vi "Main.vi"() -> ()   [LabVIEW 2019]
doc: "This Continuous Measurement sample project is based on the Queued Message Handler template.\n\nThe Event Handling Loop generates messages based on user interface actions.\n\nThe Message Handling Loop processes messages generated by the Event Handling Loop, or by other messages. There are also Acquisition and Logging message handling loop subVIs, and a chart updating loop."
uses:
  Settings/Settings.ctl
  HardwareAdapter/Support/Hardware Configuration.ctl
  HardwareAdapter/Support/Camera Configuration.ctl
  D:/SDK/PMQI-LabViewSamples/Examples/Dependencies/PVCamNET.dll
  <vilib>/userdefined/High Color/IMAQdx.ctl
  E:/DevHardSoftware/MMicroscopy/HardwareAdapter/Lasers/Dependencies/Oxxius_Boxx.dll
  HardwareAdapter/Lasers/Dependencies/Oxxius_Boxx.dll
  Logging/Logging Configuration.ctl
  controls/UI Configuration.ctl
  controls/CallBack Refs.ctl
  controls/UI Data.ctl
  controls/UI State.ctl
  controls/ImageInfo.ctl
  <vilib>/vision/Image Controls.llb/IMAQ Image.ctl
  HardwareAdapter/Lasers/Laser Ctrl.ctl
  HardwareAdapter/Stages/Stage Ctrl.ctl
  Global.vi
  support/Message Queue/Enqueue Message (Single).vi
  <vilib>/Utility/error.llb/Error Cluster From Error Code.vi
  <vilib>/ErrorRing/Error Ring.xnode
  Acquisition/Acquisition.lvlib
  Logging/Logging.lvlib
  Settings/Settings.lvlib
  support/User Event - Stop/User Event - Stop.lvlib
  support/Message Queue/Message Queue.lvlib
  Settings/Settings Dialog.vi
panel:
  in  "DropFrame":dbl
  in  "FrameIndexSroll":i32(c297)
  in  "RealFPS":dbl
  in  "FrameRate":dbl
  in  "CaptureFrame":dbl
  in  "Exposure":dbl
  in  "CurrentFrame":dbl
  out "CapturingLED":bool caption="Capturing"
  in  "TableTap":T1(tab)
  out "8 Bit Histogram":u32[](graph)
  out "EPILimit":bool
  out "TIRFLimit":bool
  in  "MicroStage+":dbl
  in  "TIRF-":bool
  in  "TIRF--":bool
  in  "EPI++":bool
  in  "EPI+":bool
  out "TirfModuleScollBar":u8(slide) scale=0.0..100.0
  in  "Anti-Drifft XY":bool
  out "NanoStage X":dbl(graph)
  out "NanoStage  Y":dbl(graph)
  out "NanoStage Z":dbl(graph)
  out "TIRF-Lock":cluster{"X":dbl, "Y":dbl}[](graph)
  in  "TIRF-Lock Z":bool
  in  "StageX-":bool
  in  "StageX+":bool
  in  "StageY+":bool
  in  "StageY-":bool
  in  "StageZ++":bool
  in  "StageZ--":bool
  in  "StageY++":bool
  in  "StageZ+":bool
  in  "StageZ-":bool
  in  "StageX--":bool
  in  "StageX++":bool
  in  "StageY--":bool
  in  "XYIncreatement+":dbl
  in  "XYIncreatement++":dbl
  in  "ZIncreatement+":dbl
  in  "ZIncreatement++":dbl
  in  "TIRF-LockCalbrate":bool
  out "Min":u32
  out "Max":u32
  out "Mean":dbl
  in  "FileSaveButton":bool
  in  "NoteAutoSave":bool caption="AutoSave"
  in  "Note":string
  in  "FilePrefix":string
  in  "Config":T2 {"Hardware Configuration"."Lasers Configuration"."SettingValues"."785 Power" format="%.1f"; "Hardware Configuration"."Lasers Configuration"."SettingValues"."647 Power" format="%.1f"; "Hardware Configuration"."Lasers Configuration"."SettingValues"."561 Power" format="%.1f"; "Hardware Configuration"."Lasers Configuration"."SettingValues"."532 Power" format="%.1f"; "Hardware Configuration"."Lasers Configuration"."SettingValues"."488 Power" format="%.1f"; "Hardware Configuration"."Lasers Configuration"."SettingValues"."405 Power" format="%.1f"}
  in  "Save Settings":bool
  in  "AutoFocus":bool
  in  "AddROI":bool
  in  "Record":bool
  in  "Power785":dbl
  in  "785 nm":bool
  in  "Power647":sgl
  in  "647 nm":bool
  in  "Power561":dbl
  in  "561 nm":bool
  in  "Power532":sgl
  in  "532 nm":bool
  in  "Power488":dbl
  in  "488 nm":bool
  in  "Power405":dbl
  in  "405 nm":bool
  out "DeviceStatus":T9
  out "Status":string
  in  "Exit":bool
  in  "Settings":bool
  in  "Stop":bool
  in  "Album":bool
  out "RecordLED":bool caption="Rec"
  out "LiveLED":bool caption="Live"
  out "RawImage":T10(plugin-control)
  # "Power(%)"
  # "On"
  # "Off"
  # "Lasers"
  # "Y"
  # "μm"
  # "μm"
  # "μm"
  # "μm"
  # "X"
  # "TIRF"
  # "EPI"
  # "Z"
  # "μm"
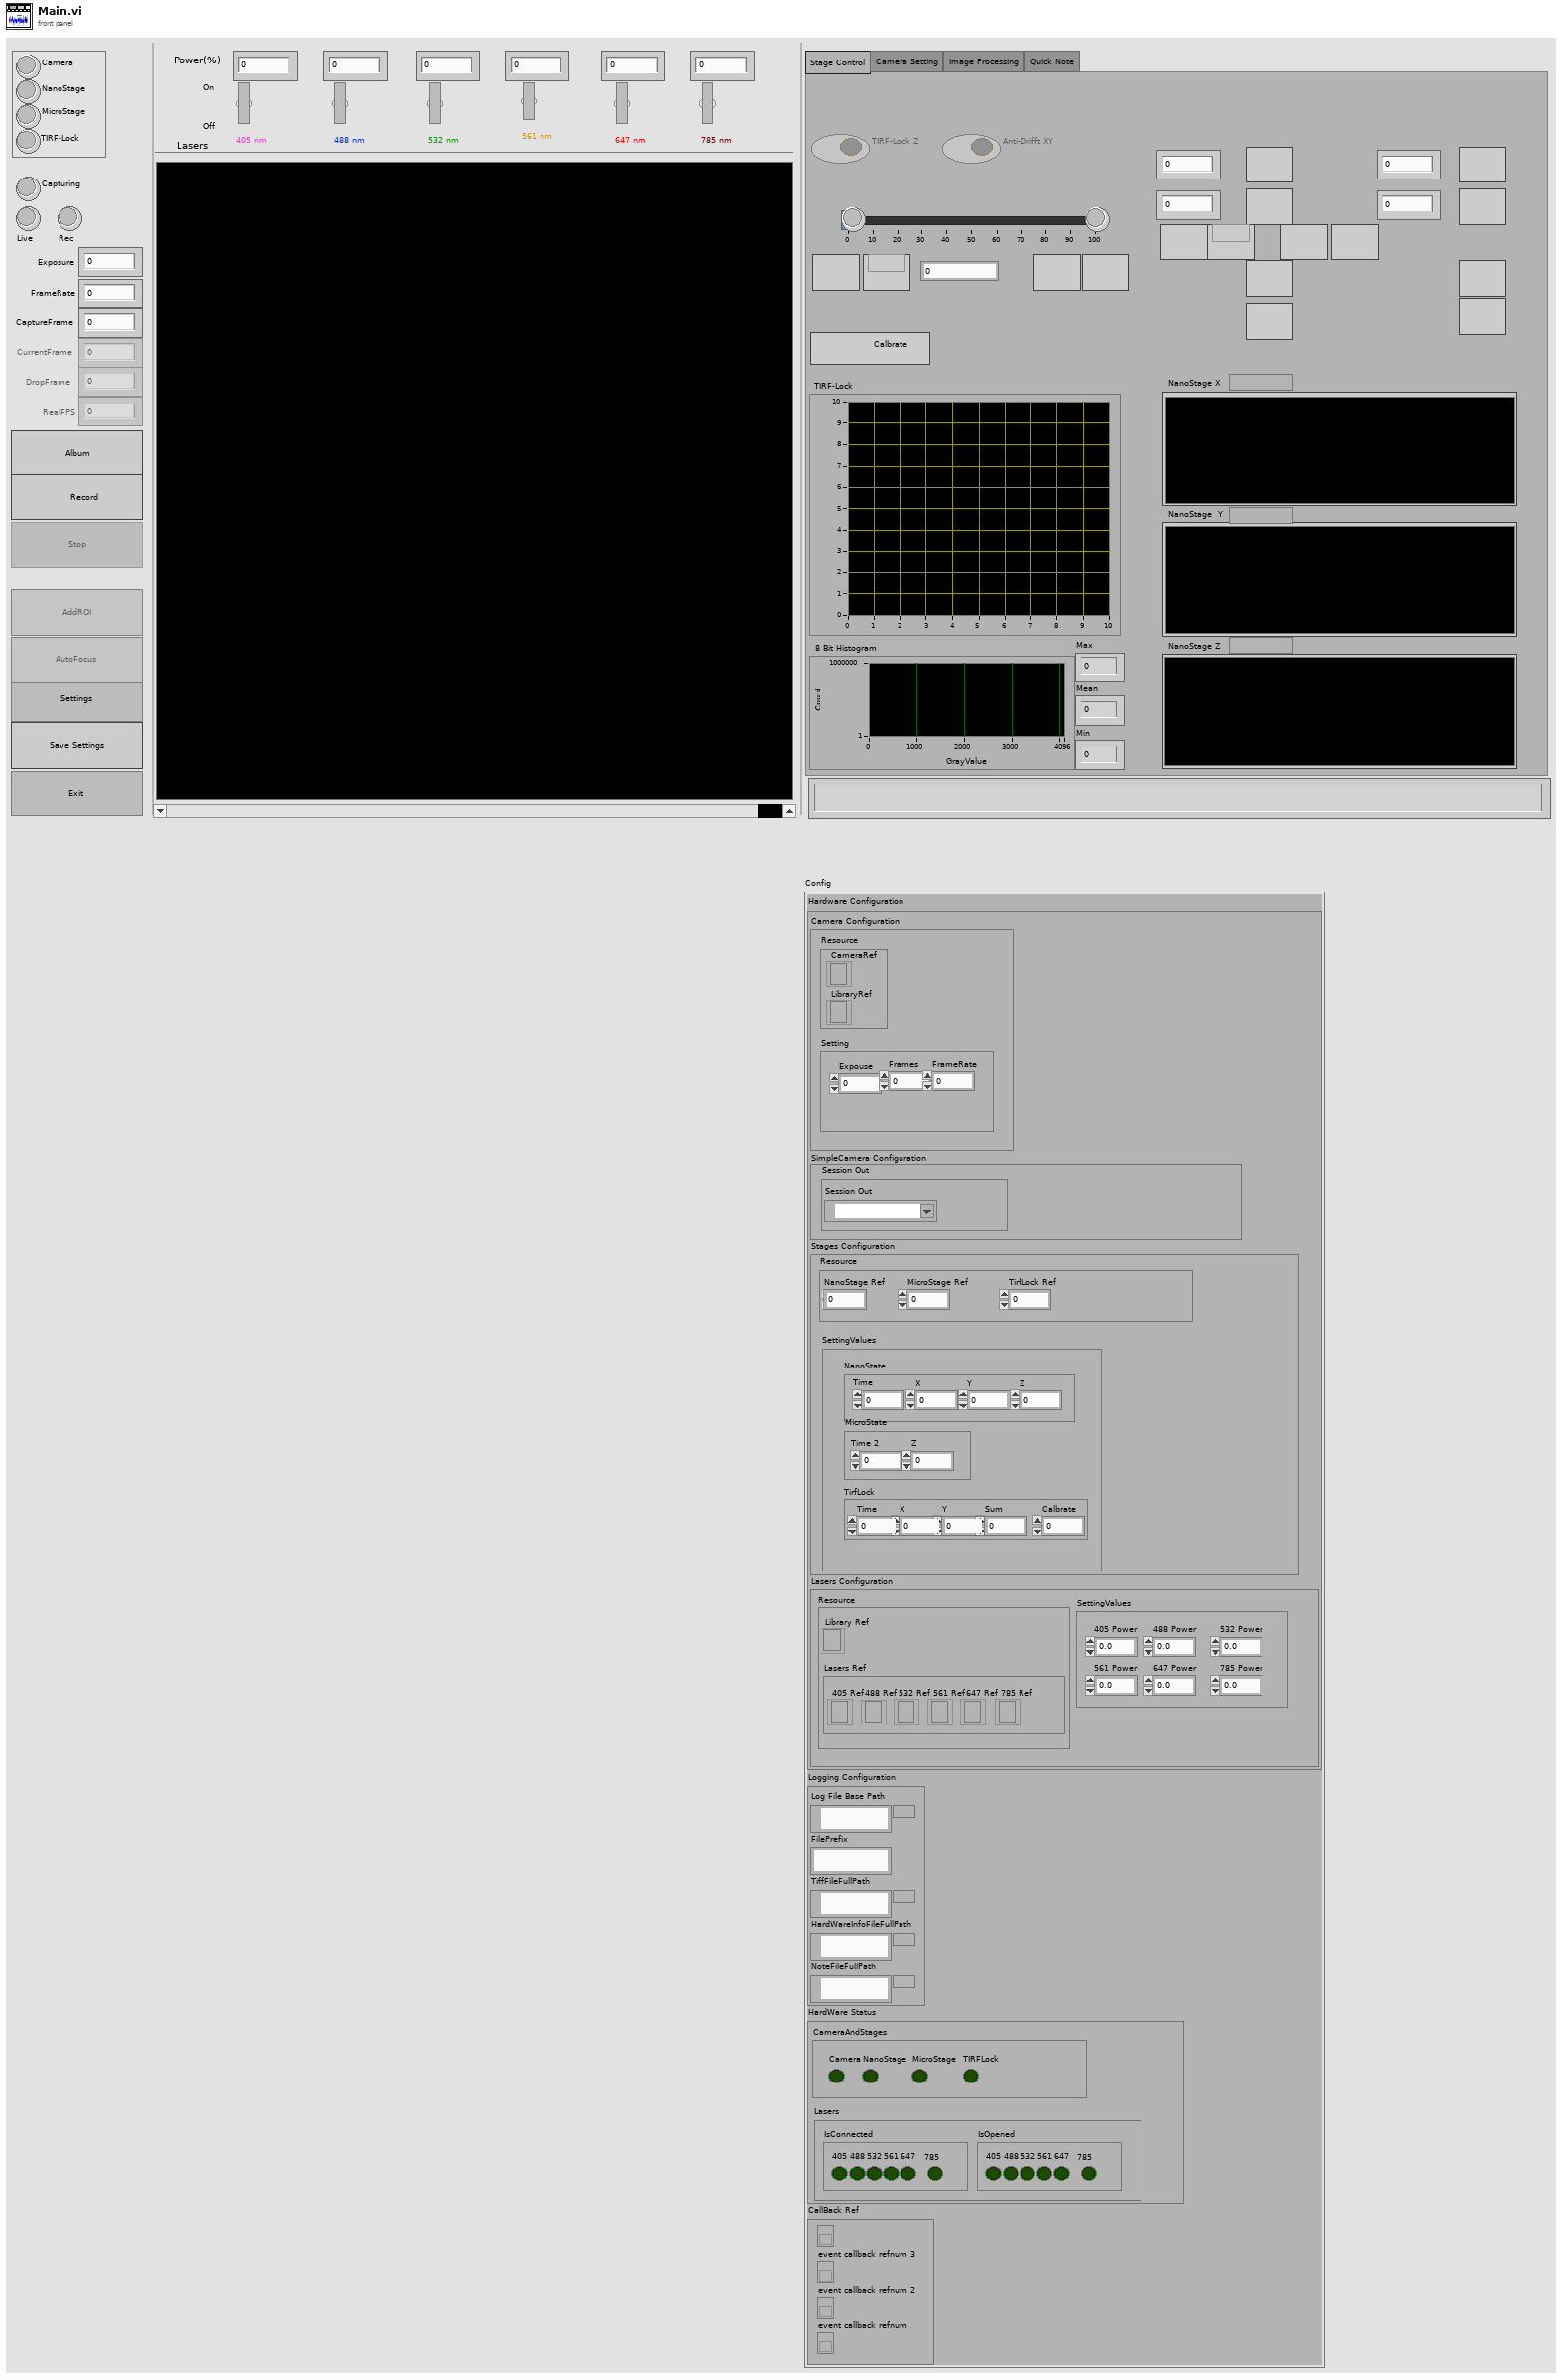
[diagram p1: front panel]
types:
  T1 = enum32{"Stage Control", "Camera Setting", "Image Processing", "Quick Note"}
  T2 = typedef "Settings.lvlib/Settings.ctl" = cluster{"Hardware Configuration":T3, "Logging Configuration":T6, "HardWare Status":cluster{"CameraAndStages":T7, "Lasers":cluster{"IsConnected":cluster{"405":bool, "488":bool, "532":bool, "561":bool, "647":bool, "785":bool}, "IsOpened":cluster{"405":bool, "488":bool, "532":bool, "561":bool, "647":bool, "785":bool}}}, "CallBack Ref":T8}
  T3 = typedef "Hardware Configuration.ctl" = cluster{"Camera Configuration":T4, "SimpleCamera Configuration":cluster{"Resource":cluster{"Session Out":T5}}, "Stages Configuration":cluster{"Resource":cluster{"NanoStage Ref":i32, "MicroStage Ref":i32, "TirfLock Ref":i32}, "SettingValues":cluster{"NanoState":cluster{"Time":dbl, "X":dbl, "Y":dbl, "Z":dbl}, "MicroState":cluster{"Time 2":dbl, "Z":dbl}, "TirfLock":cluster{"Time":dbl, "X":dbl, "Y":dbl, "Sum":dbl, "Calbrate":dbl}}}, "Lasers Configuration":cluster{"SettingValues":cluster{"405 Power":sgl, "488 Power":sgl, "532 Power":sgl, "561 Power":sgl, "647 Power":sgl, "785 Power":sgl}, "Resource":cluster{"Library Ref":refnum<k24>, "Lasers Ref":cluster{"405 Ref":refnum<k24>, "488 Ref":refnum<k24>, "532 Ref":refnum<k24>, "561 Ref":refnum<k24>, "647 Ref":refnum<k24>, "785 Ref":refnum<k24>}}}}
  T4 = typedef "Camera Configuration.ctl" = cluster{"Resource":cluster{"CameraRef":refnum<k24>, "LibraryRef":refnum<k24>}, "Setting":cluster{"Expouse":dbl, "Frames":dbl, "FrameRate":dbl}}
  T5 = typedef "IMAQdx.ctl" = refnum<k21>
  T6 = typedef "Logging.lvlib/Logging Configuration.ctl" = cluster{"Log File Base Path":path, "FilePrefix":string, "TiffFileFullPath":path, "HardWareInfoFileFullPath":path, "NoteFileFullPath":path}
  T7 = typedef "UI Configuration.ctl" = cluster{"Camera":bool, "NanoStage":bool, "MicroStage":bool, "TIRFLock":bool}
  T8 = typedef "CallBack Refs.ctl" = cluster{"event callback refnum":refnum<k27>, "event callback refnum 2":refnum<k27>, "event callback refnum 3":refnum<k27>, "event callback refnum 4":refnum<k27>}
  T9 = cluster{"Camera":bool, "NanoStage":bool, "MicroStage":bool, "TIRF-Lock":bool}
  T10 = typedef "IMAQ Image.ctl" = refnum<image>
  T11 = typedef "UI State.ctl" = enum16{"Idle", "Acquiring and Logging", "Waiting for Exit", "Waiting for Exit (Acq Stopped)", "Waiting for Exit (Ctrl Stopped)", "Waiting for Exit (Log Stopped)", "Waiting for Stop", "Waiting for Stop (Acq Stopped)", "Waiting for Stop (Ctrl Stopped)", "Waiting for Stop (Log Stopped)"}
  T12 = typedef "UI Data.ctl" = cluster{"Album Ref":refnum<vi>, "Stop Ref":refnum<vi>, "Settings Ref":refnum<vi>, "Exit Ref":refnum<vi>, "Status Ref":refnum<vi>, "Record Ref":refnum<vi>, "785 Ref":refnum<vi>, "647 Ref":refnum<vi>, "532 Ref":refnum<vi>, "561 Ref":refnum<vi>, "488 Ref":refnum<vi>, "405 Ref":refnum<vi>, "Power561 Ref":refnum<vi>, "Power405 Ref":refnum<vi>, "Power488 Ref":refnum<vi>, "Power785 Ref":refnum<vi>, "Power532 Ref":refnum<vi>, "Power647 Ref":refnum<vi>, "TIRFLock Ref":refnum<vi>, "AntiDrifft Ref":refnum<vi>, "Histogram":refnum<vi>, "Capturing":refnum<vi>, "FrameIndex":refnum<vi>, "RealFPS":refnum<vi>, "FrameIndexSroll":refnum<vi>, "DropFrame":refnum<vi>}
  T13 = typedef "Message Queue.lvlib/All Message Queues.ctl" = cluster{"UI":refnum<queue>, "Acquisition":refnum<queue>, "Logging":refnum<queue>, "Control":refnum<queue>}
  T14 = typedef "DataQueuesAndNotifier.ctl" = cluster{"DataQueues":refnum<queue>[], "DataNotifier":refnum<notifier>[]}
  T15 = typedef "ImageInfo.ctl" = cluster{"Time":dbl, "Image":T10, "Histogram":u32[], "MeanValue":dbl, "Min":u32, "Max":u32}
  T16 = typedef "LVPoint32TypeDef.ctl" = cluster{"Horizontal":i32, "Vertical":i32}
  T17 = typedef "Laser Ctrl.ctl" = cluster{"Laser Ref":refnum<k24>, "statue":bool, "Power":dbl, "Power Ref":refnum<vi>}
  T18 = typedef "Stage Ctrl.ctl" = cluster{"Axis":dbl, "value":dbl, "direction":bool}
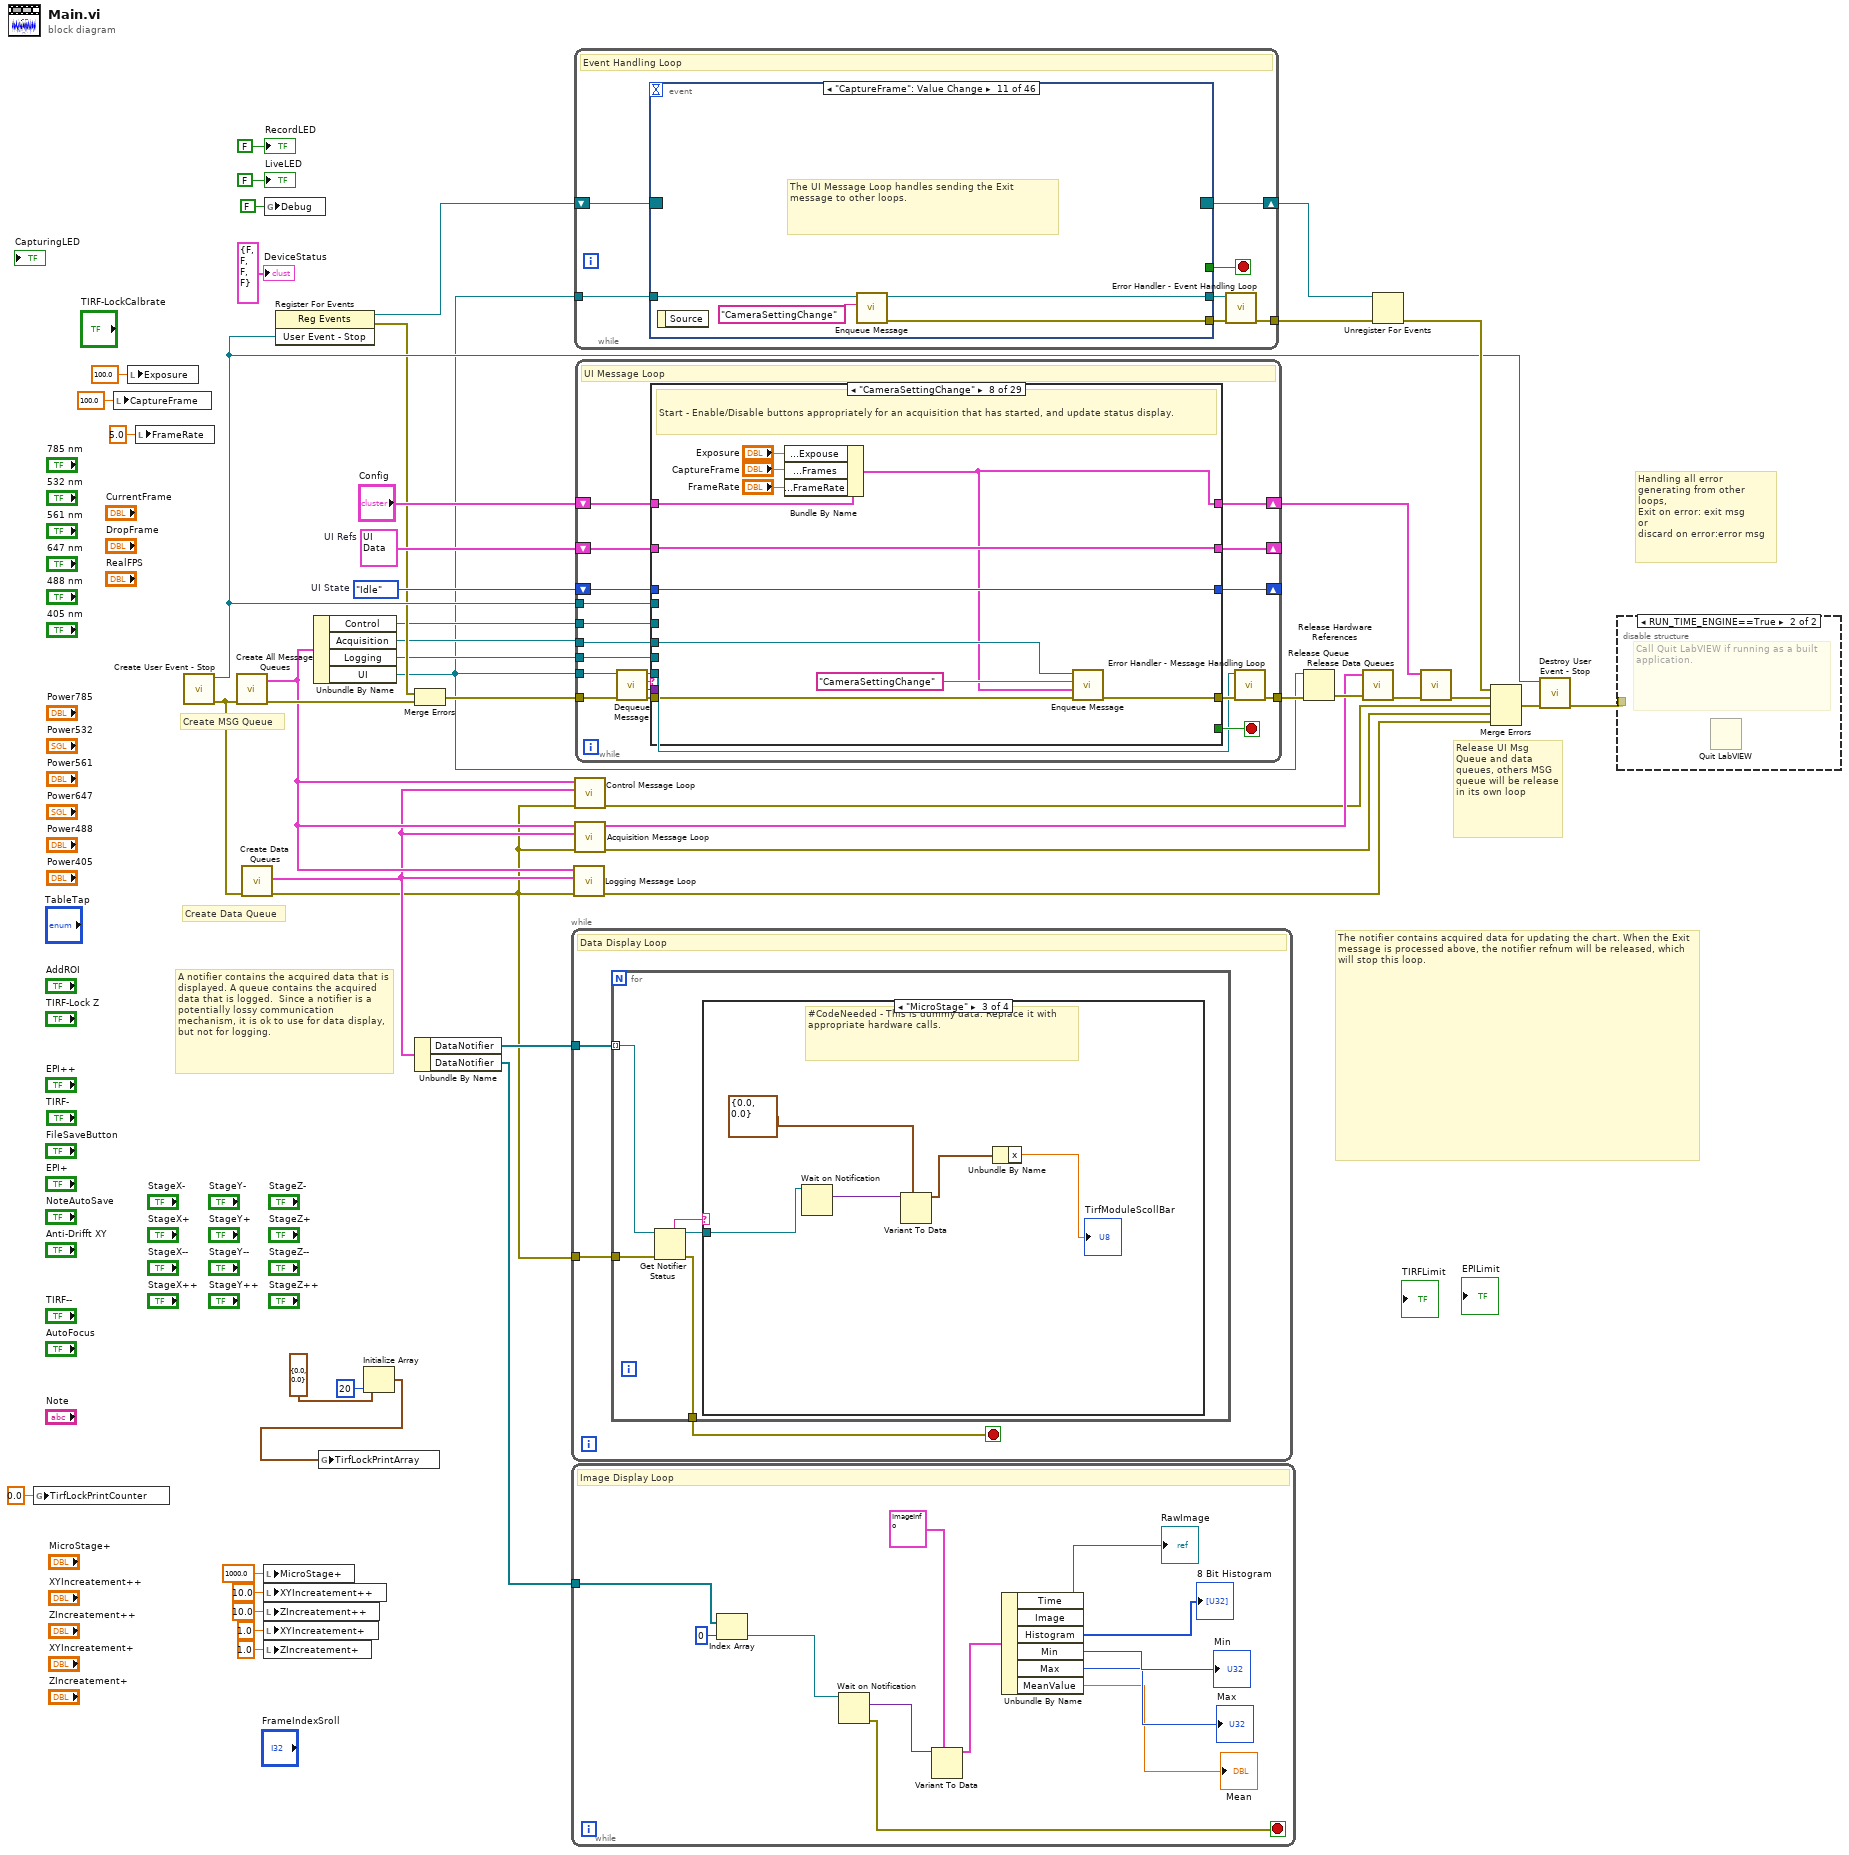
[diagram p0: block diagram]
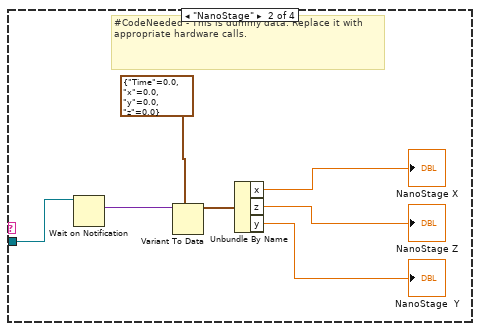
[diagram p4: hidden frame]
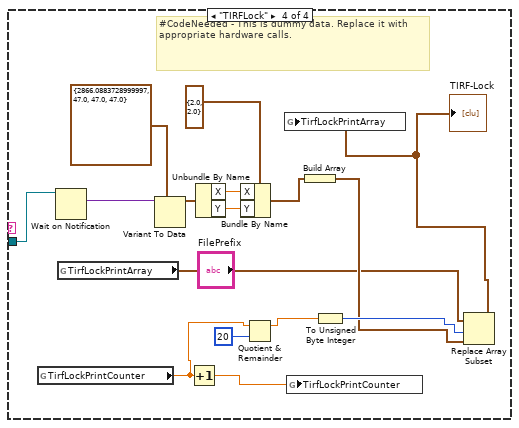
[diagram p5: hidden frame]
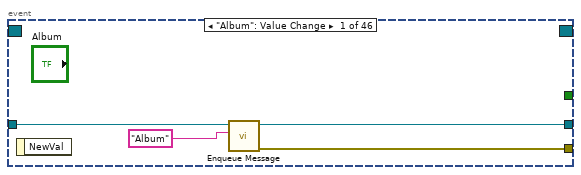
[diagram p6: hidden frame]
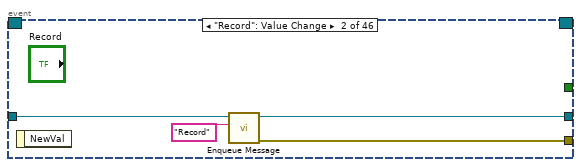
[diagram p7: hidden frame]
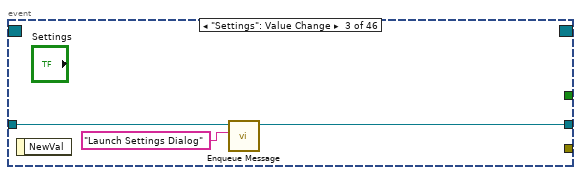
[diagram p8: hidden frame]
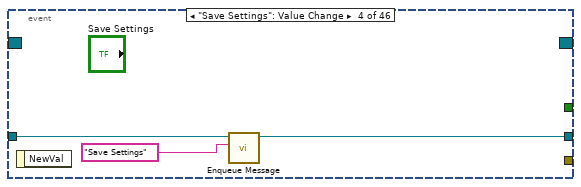
[diagram p9: hidden frame]
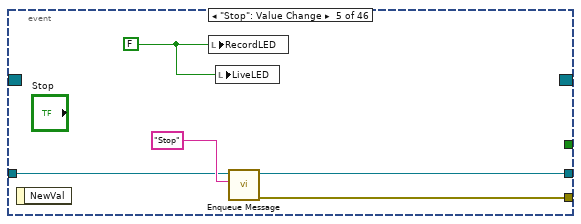
[diagram p10: hidden frame]
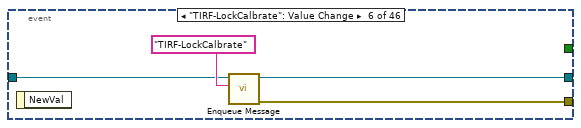
[diagram p11: hidden frame]
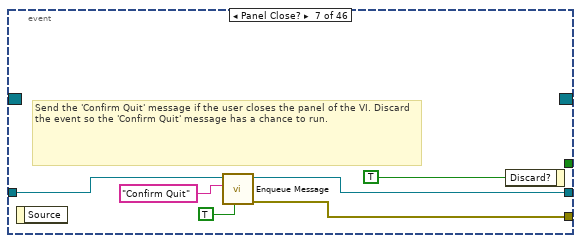
[diagram p12: hidden frame]
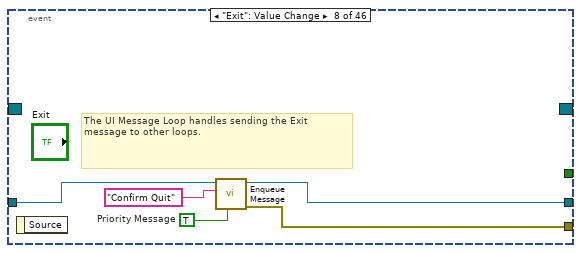
[diagram p13: hidden frame]
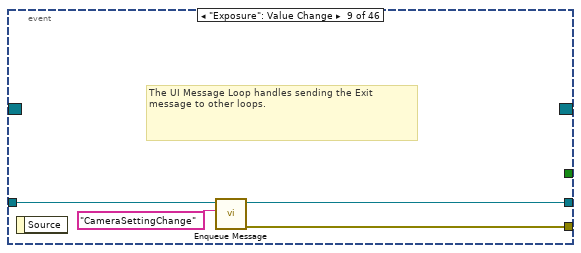
[diagram p14: hidden frame]
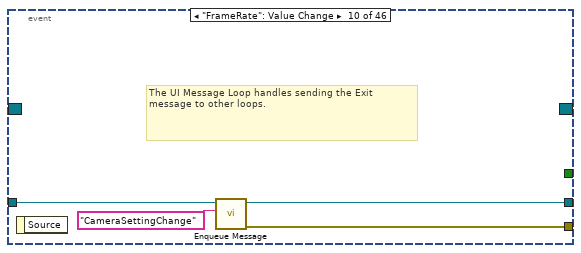
[diagram p15: hidden frame]
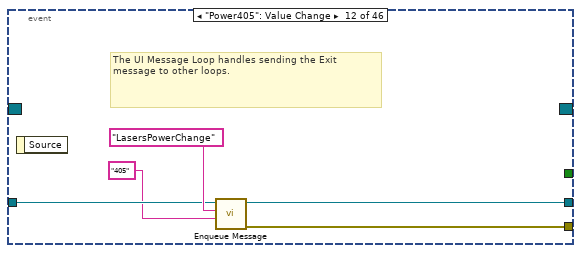
[diagram p16: hidden frame]
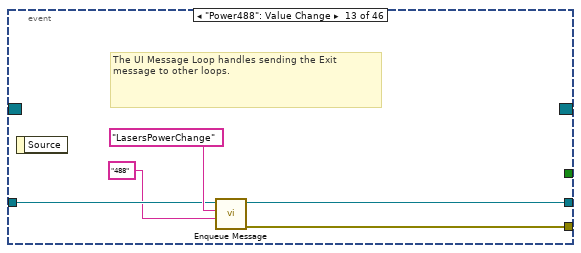
[diagram p17: hidden frame]
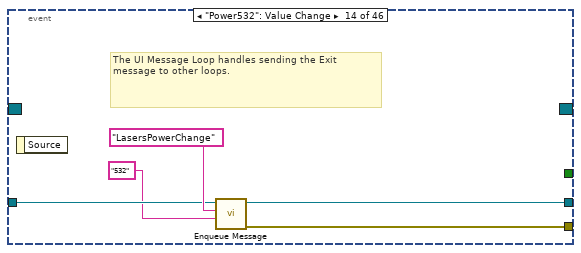
[diagram p18: hidden frame]
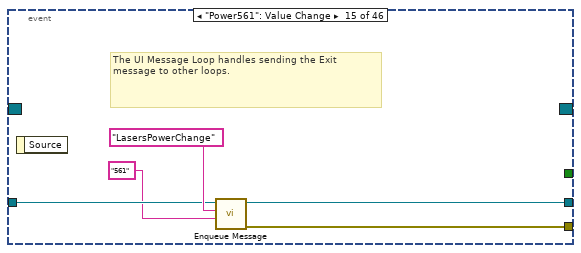
[diagram p19: hidden frame]
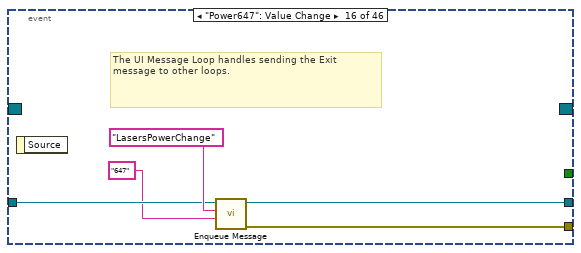
[diagram p20: hidden frame]
diagram:
  w42 = UI_State."Idle"  # UI State
  w43 = T12 {"Album Ref"=refnum, "Stop Ref"=refnum, "Settings Ref"=refnum, "Exit Ref"=refnum, "Status Ref"=refnum, "Record Ref"=refnum, "785 Ref"=refnum, "647 Ref"=refnum, "532 Ref"=refnum, "561 Ref"=refnum, "488 Ref"=refnum, "405 Ref"=refnum, "Power561 Ref"=refnum, "Power405 Ref"=refnum, "Power488 Ref"=refnum, "Power785 Ref"=refnum, "Power532 Ref"=refnum, "Power647 Ref"=refnum, "TIRFLock Ref"=refnum, "AntiDrifft Ref"=refnum, "Histogram"=refnum, "Capturing"=refnum, "FrameIndex"=refnum, "RealFPS"=refnum, "FrameIndexSroll"=refnum, "DropFrame"=refnum}  # UI Refs
  # "Create Data Queue"
  # "Create MSG Queue"
  # "Handling all error\ngenerating from other \nloops,\nExit on error: exit msg\nor\ndiscard on error:error msg"
  # "Release UI Msg Queue and data queues, others MSG queue will be release in its own loop"
  # "A notifier contains the acquired data that is displayed. A queue contains the acquired data that is logged.  Since a notifier is a potentially lossy communication mechanism, it is ok to use for data display, but not for logging."
  # "The notifier contains acquired data for updating the chart. When the Exit message is processed above, the notifier refnum will be released, which will stop this loop."
  n1 = global write "Global.vi" "TirfLockPrintCounter"(0.0 ("TirfLockPrintCounter")) -> ()
  n2 = local write "CaptureFrame"(100.0 ("CaptureFrame")) -> ()
  n3 = local write "Exposure"(100.0 ("Exposure")) -> ()
  n4 = local write "FrameRate"(5.0 ("FrameRate")) -> ()
  n5 = call "Create User Event - Stop.vi"() -> ("error out"=w11:errorcluster, "User Event - Stop"=w38:refnum<user-event>)  [unwired: 10 in]
  n6 = call "Create All Message Queues.vi"("error in (no error)"=w11) -> ("error out"=w35:errorcluster, "Message Queues out"=w22:T13)  [unwired: 9 in]
  n7 = call "Create Data Queues.vi"("error in (no error)"=w11) -> ("error out"=w15:errorcluster, "DataQueuesAndNotifier Out"=w17:T14)  [unwired: 9 in]
  n8 = local write "MicroStage+"(1000.0 ("MicroStage+")) -> ()
  n9 = local write "XYIncreatement++"(10.0 ("XYIncreatement++")) -> ()
  n10 = local write "ZIncreatement++"(10.0 ("ZIncreatement++")) -> ()
  n11 = local write "XYIncreatement+"(1.0 ("XYIncreatement+")) -> ()
  n12 = local write "ZIncreatement+"(1.0 ("ZIncreatement+")) -> ()
  n13 = global write "Global.vi" "Debug"(FALSE ("Debug")) -> ()
  n14 = register-events(w38) -> (reference out=w39:refnum<event-registration>, error out=w36:errorcluster)  [unwired: 2 in]
  n15 = Unbundle By Name(w22) -> ("Control"=w24:refnum<queue>, "Acquisition"=w26:refnum<queue>, "Logging"=w25:refnum<queue>, "UI"=w23:refnum<queue>)
  n16 = Initialize Array(cluster{"X":dbl, "Y":dbl} {"X"=0.0, "Y"=0.0} ("TirfLock"), 20 ("dimension size")) -> (w27:cluster{"X":dbl, "Y":dbl}[])
  n17 = global write "Global.vi" "TirfLockPrintArray"(w27) -> ()
  n18 = Merge Errors(w36, w35) -> (w37:errorcluster)
  n19 = Unbundle By Name(w17) -> ("DataNotifier"=w16:refnum<notifier>[], "DataNotifier"=w5:refnum<notifier>[])
  n20 = while "Data Display Loop" {
    tunnel: w16 -> [w49]
    tunnel: w15 -> [w50]
    stop <- w51 stop-if-true
    # "Data Display Loop"
    n21 = for {
      tunnel: [w55] -> w51
      tunnel: w49 -> [w54] mode=indexing
      tunnel: w50 -> [w53]
      n22 = Get Notifier Status(notifier=w54, error in (no error)=w53) -> (notifier out=w52:refnum<notifier>, notifier name=w56:string, error out=w55:errorcluster)  [unwired: 2 out]
      n23 = case shown="\"MicroStage\"" w56 {
        tunnel: w52 -> [_ w57 w64 w69]
        frame Default {
        }
        frame "NanoStage" {
          # "#CodeNeeded - This is dummy data. Replace it with appropriate hardware calls."
          n24 = Wait on Notification(notifier=w57) -> (notification=w63:variant)  [unwired: 3 in, 3 out]
          n25 = Variant To Data(type=cluster{"Time":dbl, "x":dbl, "y":dbl, "z":dbl} {"Time"=0.0, "x"=0.0, "y"=0.0, "z"=0.0} ("NanoStage"), Variant=w63) -> (data=w61:cluster{"Time":dbl, "x":dbl, "y":dbl, "z":dbl})  [unwired: 1 in, 1 out]
          n26 = Unbundle By Name(w61) -> ("x"=→"NanoStage X":dbl, "z"=→"NanoStage Z":dbl, "y"=→"NanoStage  Y":dbl)
        }
        frame "MicroStage" {
          # "#CodeNeeded - This is dummy data. Replace it with appropriate hardware calls."
          n27 = Wait on Notification(notifier=w64) -> (notification=w68:variant)  [unwired: 3 in, 3 out]
          n28 = Variant To Data(type=cluster{"Time":dbl, "x":dbl} {"Time"=0.0, "x"=0.0} ("NanoStage"), Variant=w68) -> (data=w66:cluster{"Time":dbl, "x":dbl})  [unwired: 1 in, 1 out]
          n29 = Unbundle By Name(w66) -> ("x"=→"TirfModuleScollBar":dbl)
        }
        frame "TIRFLock" {
          # "#CodeNeeded - This is dummy data. Replace it with appropriate hardware calls."
          n30 = global read "Global.vi" "TirfLockPrintCounter"() -> (w72:dbl)
          n31 = Wait on Notification(notifier=w69) -> (notification=w84:variant)  [unwired: 3 in, 3 out]
          n32 = global read "Global.vi" "TirfLockPrintArray"() -> (w71:cluster{"X":dbl, "Y":dbl}[])
          n33 = Variant To Data(type=cluster{"Time":dbl, "X":dbl, "Y":dbl, "Sum":dbl} {"Time"=2866.0883728999997, "X"=47.0, "Y"=47.0, "Sum"=47.0} ("TirfLock"), Variant=w84) -> (data=w82:cluster{"Time":dbl, "X":dbl, "Y":dbl, "Sum":dbl})  [unwired: 1 in, 1 out]
          n34 = Increment(x=w72) -> (x+1=w75:dbl)
          n35 = Unbundle By Name(w82) -> ("X"=w80:dbl, "Y"=w79:dbl)
          n36 = Bundle By Name(cluster=cluster{"X":dbl, "Y":dbl} {"X"=2.0, "Y"=2.0} ("TirfLock"), "X"=w80, "Y"=w79) -> (w76:cluster{"X":dbl, "Y":dbl})
          n37 = Quotient & Remainder(x=w72, y=20) -> (x-y*floor(x/y)=w77:dbl)  [unwired: 1 out]
          n38 = global write "Global.vi" "TirfLockPrintCounter"(w75) -> ()
          n39 = Build Array(w76) -> (w73:cluster{"X":dbl, "Y":dbl}[])
          n40 = To Unsigned Byte Integer(number=w77) -> (unsigned 8bit integer=w74:u8)
          n41 = Replace Array Subset(array=w71, new element=w73, index=w74) -> (w70:cluster{"X":dbl, "Y":dbl}[])
          "TIRF-Lock" <- w70
          n42 = global write "Global.vi" "TirfLockPrintArray"(w70) -> ()
        }
      }
    }
  }
  n43 = while {
    tunnel: w5 -> [w96]
    stop <- w90 stop-if-true
    # "Image Display Loop"
    n44 = Index Array(array=w96, index=0) -> (element=w91:refnum<notifier>)
    n45 = Wait on Notification(notifier=w91) -> (notification=w89:variant, error out=w90:errorcluster)  [unwired: 3 in, 2 out]
    n46 = Variant To Data(type=T15 {"Time"=0.0, "Image"=refnum, "Histogram"=[], "MeanValue"=0.0, "Min"=0, "Max"=0} ("RawImage"), Variant=w89) -> (data=w95:T15)  [unwired: 1 in, 1 out]
    n47 = Unbundle By Name(w95) -> ("Image"=→"RawImage":T10, "Histogram"=→"8 Bit Histogram":u32[], "Min"=→"Min":u32, "Max"=→"Max":u32, "MeanValue"=→"Mean":dbl)  [unwired: 1 out]
  }
  n48 = call "Logging Message Loop.vi"("error in (no error)"=w15, "DataQueuesAndNotifier"=w17, "Message Queues"=w22) -> ("error out"=w20:errorcluster)  [unwired: 8 in]
  n49 = while {
    tunnel: w23 -> [w102]
    tunnel: [w99] -> w47
    shift-right: [w101] -> w44
    shift-left: w39 -> [w103]
    stop <- w100 stop-if-true
    # "Event Handling Loop"
    n50 = event shown="[10] \"CaptureFrame\": Value Change" {
      selector: w103 -> [_ _ _ _ _ _ _ _ _ _ _ _ _ _ _ _ _ _ _ _ _ _ _ _ _ _ _ _ _ _ _ _ _ _ _ _ _ _ _ _ _ _ _ _ _ _]
      dyn-events: [_ _ _ _ _ _ _ _ _ _ _ _ _ _ _ _ _ _ _ _ _ _ _ _ _ _ _ _ _ _ _ _ _ _ _ _ _ _ _ _ _ _ _ _ _ _] -> w101
      timeout: _ -> [_ _ _ _ _ _ _ _ _ _ _ _ _ _ _ _ _ _ _ _ _ _ _ _ _ _ _ _ _ _ _ _ _ _ _ _ _ _ _ _ _ _ _ _ _ _]
      tunnel: [_ _ _ _ _ _ _ _ _ _ _ _ _ _ _ _ _ _ _ _ _ _ _ _ _ _ _ _ _ _ _ _ _ _ _ _ _ _ _ _ _ _ _ _ _ TRUE ("Discard?")] -> w100
      tunnel: w102 -> [w107 w111 w113 w116 w121 w125 w130 w134 w139 w143 w147 w152 w157 w162 w167 w172 w177 w182 w187 w192 w197 w202 w207 w212 w217 w222 w227 w232 w237 w242 w247 w252 w257 w262 w267 w272 w277 w282 w287 w292 w299 w308 w314 w316 w320 w324]
      tunnel: [w105 w109 _ _ w120 w124 w128 w137 w141 w145 w149 w154 w159 w164 w169 w174 w179 w184 w189 w194 w199 w204 w209 w214 w219 w224 w229 w234 w239 w244 w249 w254 w259 w264 w269 w274 w279 w284 w289 w294 _ w310 _ _ w323 _] -> w98
      tunnel: [w104 w108 w112 w115 w119 w123 w129 w133 w138 w142 w146 w151 w156 w161 w166 w171 w176 w181 w186 w191 w196 w201 w206 w211 w216 w221 w226 w231 w236 w241 w246 w251 w256 w261 w266 w271 w276 w281 w286 w291 w299 w307 w314 w316 w319 w324] -> w97
      event "Album": Value Change {
        n51 = event-data() -> ()  [unwired: 1 in, 1 out]
        n52 = call-poly "Enqueue Message.vi"("Message"="Album", "Message Queue"=w107) -> ("error out"=w105:errorcluster, "dup Message Queue"=w104:refnum<queue>)  [unwired: 8 in]
      }
      event "Record": Value Change {
        n53 = event-data() -> ()  [unwired: 1 in, 1 out]
        n54 = call-poly "Enqueue Message.vi"("Message"="Record", "Message Queue"=w111) -> ("error out"=w109:errorcluster, "dup Message Queue"=w108:refnum<queue>)  [unwired: 8 in]
      }
      event "Settings": Value Change {
        n55 = event-data() -> ()  [unwired: 1 in, 1 out]
        n56 = call-poly "Enqueue Message.vi"("Message"="Launch Settings Dialog", "Message Queue"=w113) -> ("dup Message Queue"=w112:refnum<queue>)  [unwired: 8 in, 1 out]
      }
      event "Save Settings": Value Change {
        n57 = event-data() -> ()  [unwired: 1 in, 1 out]
        n58 = call-poly "Enqueue Message.vi"("Message"="Save Settings", "Message Queue"=w116) -> ("dup Message Queue"=w115:refnum<queue>)  [unwired: 8 in, 1 out]
      }
      event "Stop": Value Change {
        w118 = FALSE ("RecordLED")
        n59 = event-data() -> ()  [unwired: 1 in, 1 out]
        n60 = local write "RecordLED"(w118) -> ()
        n61 = local write "LiveLED"(w118) -> ()
        n62 = call-poly "Enqueue Message.vi"("Message"="Stop", "Message Queue"=w121) -> ("error out"=w120:errorcluster, "dup Message Queue"=w119:refnum<queue>)  [unwired: 8 in]
      }
      event "TIRF-LockCalbrate": Value Change {
        n63 = event-data() -> ()  [unwired: 1 in, 1 out]
        n64 = call-poly "Enqueue Message.vi"("Message"="TIRF-LockCalbrate", "Message Queue"=w125) -> ("error out"=w124:errorcluster, "dup Message Queue"=w123:refnum<queue>)  [unwired: 8 in]
      }
      event Panel Close? {
        # "Send the 'Confirm Quit' message if the user closes the panel of the VI. Discard the event so the 'Confirm Quit' message has a chance to run."
        n65 = event-data() -> ()  [unwired: 1 in, 1 out]
        n66 = call-poly "Enqueue Message.vi"("Priority Message? (F)"=TRUE, "Message"="Confirm Quit", "Message Queue"=w130) -> ("error out"=w128:errorcluster, "dup Message Queue"=w129:refnum<queue>)  [unwired: 7 in]
        n67 = event-data("Discard?"=TRUE) -> ()  [unwired: 1 in, 1 out]
      }
      event "Exit": Value Change {
        w135 = TRUE  # Priority Message
        # "The UI Message Loop handles sending the Exit message to other loops."
        n68 = event-data() -> ()  [unwired: 1 in, 1 out]
        n69 = call-poly "Enqueue Message.vi"("Priority Message? (F)"=w135, "Message"="Confirm Quit", "Message Queue"=w134) -> ("error out"=w137:errorcluster, "dup Message Queue"=w133:refnum<queue>)  [unwired: 7 in]
      }
      event "Exposure": Value Change {
        # "The UI Message Loop handles sending the Exit message to other loops."
        n70 = event-data() -> ()  [unwired: 1 in, 1 out]
        n71 = call-poly "Enqueue Message.vi"("Message"="CameraSettingChange", "Message Queue"=w139) -> ("error out"=w141:errorcluster, "dup Message Queue"=w138:refnum<queue>)  [unwired: 8 in]
      }
      event "FrameRate": Value Change {
        # "The UI Message Loop handles sending the Exit message to other loops."
        n72 = event-data() -> ()  [unwired: 1 in, 1 out]
        n73 = call-poly "Enqueue Message.vi"("Message"="CameraSettingChange", "Message Queue"=w143) -> ("error out"=w145:errorcluster, "dup Message Queue"=w142:refnum<queue>)  [unwired: 8 in]
      }
      event "CaptureFrame": Value Change {
        # "The UI Message Loop handles sending the Exit message to other loops."
        n74 = event-data() -> ()  [unwired: 1 in, 1 out]
        n75 = call-poly "Enqueue Message.vi"("Message"="CameraSettingChange", "Message Queue"=w147) -> ("error out"=w149:errorcluster, "dup Message Queue"=w146:refnum<queue>)  [unwired: 8 in]
      }
      event "Power405": Value Change {
        # "The UI Message Loop handles sending the Exit message to other loops."
        n76 = event-data() -> ()  [unwired: 1 in, 1 out]
        n77 = call-poly "Enqueue Message.vi"("Message Data"="405" ("Message"), "Message"="LasersPowerChange", "Message Queue"=w152) -> ("error out"=w154:errorcluster, "dup Message Queue"=w151:refnum<queue>)  [unwired: 7 in]
      }
      event "Power488": Value Change {
        # "The UI Message Loop handles sending the Exit message to other loops."
        n78 = event-data() -> ()  [unwired: 1 in, 1 out]
        n79 = call-poly "Enqueue Message.vi"("Message Data"="488" ("Message"), "Message"="LasersPowerChange", "Message Queue"=w157) -> ("error out"=w159:errorcluster, "dup Message Queue"=w156:refnum<queue>)  [unwired: 7 in]
      }
      event "Power532": Value Change {
        # "The UI Message Loop handles sending the Exit message to other loops."
        n80 = event-data() -> ()  [unwired: 1 in, 1 out]
        n81 = call-poly "Enqueue Message.vi"("Message Data"="532" ("Message"), "Message"="LasersPowerChange", "Message Queue"=w162) -> ("error out"=w164:errorcluster, "dup Message Queue"=w161:refnum<queue>)  [unwired: 7 in]
      }
      event "Power561": Value Change {
        # "The UI Message Loop handles sending the Exit message to other loops."
        n82 = event-data() -> ()  [unwired: 1 in, 1 out]
        n83 = call-poly "Enqueue Message.vi"("Message Data"="561" ("Message"), "Message"="LasersPowerChange", "Message Queue"=w167) -> ("error out"=w169:errorcluster, "dup Message Queue"=w166:refnum<queue>)  [unwired: 7 in]
      }
      event "Power647": Value Change {
        # "The UI Message Loop handles sending the Exit message to other loops."
        n84 = event-data() -> ()  [unwired: 1 in, 1 out]
        n85 = call-poly "Enqueue Message.vi"("Message Data"="647" ("Message"), "Message"="LasersPowerChange", "Message Queue"=w172) -> ("error out"=w174:errorcluster, "dup Message Queue"=w171:refnum<queue>)  [unwired: 7 in]
      }
      event "Power785": Value Change {
        # "The UI Message Loop handles sending the Exit message to other loops."
        n86 = event-data() -> ()  [unwired: 1 in, 1 out]
        n87 = call-poly "Enqueue Message.vi"("Message Data"="785" ("Message"), "Message"="LasersPowerChange", "Message Queue"=w177) -> ("error out"=w179:errorcluster, "dup Message Queue"=w176:refnum<queue>)  [unwired: 7 in]
      }
      event "405 nm": Value Change {
        # "The UI Message Loop handles sending the Exit message to other loops."
        n88 = event-data() -> ()  [unwired: 1 in, 1 out]
        n89 = call-poly "Enqueue Message.vi"("Message Data"="405" ("Message"), "Message"="LasersSwitch", "Message Queue"=w182) -> ("error out"=w184:errorcluster, "dup Message Queue"=w181:refnum<queue>)  [unwired: 7 in]
      }
      event "488 nm": Value Change {
        # "The UI Message Loop handles sending the Exit message to other loops."
        n90 = event-data() -> ()  [unwired: 1 in, 1 out]
        n91 = call-poly "Enqueue Message.vi"("Message Data"="488" ("Message"), "Message"="LasersSwitch", "Message Queue"=w187) -> ("error out"=w189:errorcluster, "dup Message Queue"=w186:refnum<queue>)  [unwired: 7 in]
      }
      event "532 nm": Value Change {
        # "The UI Message Loop handles sending the Exit message to other loops."
        n92 = event-data() -> ()  [unwired: 1 in, 1 out]
        n93 = call-poly "Enqueue Message.vi"("Message Data"="532" ("Message"), "Message"="LasersSwitch", "Message Queue"=w192) -> ("error out"=w194:errorcluster, "dup Message Queue"=w191:refnum<queue>)  [unwired: 7 in]
      }
      event "561 nm": Value Change {
        # "The UI Message Loop handles sending the Exit message to other loops."
        n94 = event-data() -> ()  [unwired: 1 in, 1 out]
        n95 = call-poly "Enqueue Message.vi"("Message Data"="561" ("Message"), "Message"="LasersSwitch", "Message Queue"=w197) -> ("error out"=w199:errorcluster, "dup Message Queue"=w196:refnum<queue>)  [unwired: 7 in]
      }
      event "647 nm": Value Change {
        # "The UI Message Loop handles sending the Exit message to other loops."
        n96 = event-data() -> ()  [unwired: 1 in, 1 out]
        n97 = call-poly "Enqueue Message.vi"("Message Data"="647" ("Message"), "Message"="LasersSwitch", "Message Queue"=w202) -> ("error out"=w204:errorcluster, "dup Message Queue"=w201:refnum<queue>)  [unwired: 7 in]
      }
      event "785 nm": Value Change {
        # "The UI Message Loop handles sending the Exit message to other loops."
        n98 = event-data() -> ()  [unwired: 1 in, 1 out]
        n99 = call-poly "Enqueue Message.vi"("Message Data"="785" ("Message"), "Message"="LasersSwitch", "Message Queue"=w207) -> ("error out"=w209:errorcluster, "dup Message Queue"=w206:refnum<queue>)  [unwired: 7 in]
      }
      event "StageX-": Value Change {
        # "The UI Message Loop handles sending the Exit message to other loops."
        n100 = event-data() -> ()  [unwired: 1 in, 1 out]
        n101 = call-poly "Enqueue Message.vi"("Message Data"="StageX-" ("Message"), "Message"="StageControlChange", "Message Queue"=w212) -> ("error out"=w214:errorcluster, "dup Message Queue"=w211:refnum<queue>)  [unwired: 7 in]
      }
      event "StageX+": Value Change {
        # "The UI Message Loop handles sending the Exit message to other loops."
        n102 = event-data() -> ()  [unwired: 1 in, 1 out]
        n103 = call-poly "Enqueue Message.vi"("Message Data"="StageX+" ("Message"), "Message"="StageControlChange", "Message Queue"=w217) -> ("error out"=w219:errorcluster, "dup Message Queue"=w216:refnum<queue>)  [unwired: 7 in]
      }
      event "StageX--": Value Change {
        # "The UI Message Loop handles sending the Exit message to other loops."
        n104 = event-data() -> ()  [unwired: 1 in, 1 out]
        n105 = call-poly "Enqueue Message.vi"("Message Data"="StageX--" ("Message"), "Message"="StageControlChange", "Message Queue"=w222) -> ("error out"=w224:errorcluster, "dup Message Queue"=w221:refnum<queue>)  [unwired: 7 in]
      }
      event "StageX++": Value Change {
        # "The UI Message Loop handles sending the Exit message to other loops."
        n106 = event-data() -> ()  [unwired: 1 in, 1 out]
        n107 = call-poly "Enqueue Message.vi"("Message Data"="StageX++" ("Message"), "Message"="StageControlChange", "Message Queue"=w227) -> ("error out"=w229:errorcluster, "dup Message Queue"=w226:refnum<queue>)  [unwired: 7 in]
      }
      event "StageY-": Value Change {
        # "The UI Message Loop handles sending the Exit message to other loops."
        n108 = event-data() -> ()  [unwired: 1 in, 1 out]
        n109 = call-poly "Enqueue Message.vi"("Message Data"="StageY-" ("Message"), "Message"="StageControlChange", "Message Queue"=w232) -> ("error out"=w234:errorcluster, "dup Message Queue"=w231:refnum<queue>)  [unwired: 7 in]
      }
      event "StageY+": Value Change {
        # "The UI Message Loop handles sending the Exit message to other loops."
        n110 = event-data() -> ()  [unwired: 1 in, 1 out]
        n111 = call-poly "Enqueue Message.vi"("Message Data"="StageY+" ("Message"), "Message"="StageControlChange", "Message Queue"=w237) -> ("error out"=w239:errorcluster, "dup Message Queue"=w236:refnum<queue>)  [unwired: 7 in]
      }
      event "StageY--": Value Change {
        # "The UI Message Loop handles sending the Exit message to other loops."
        n112 = event-data() -> ()  [unwired: 1 in, 1 out]
        n113 = call-poly "Enqueue Message.vi"("Message Data"="StageY--" ("Message"), "Message"="StageControlChange", "Message Queue"=w242) -> ("error out"=w244:errorcluster, "dup Message Queue"=w241:refnum<queue>)  [unwired: 7 in]
      }
      event "StageY++": Value Change {
        # "The UI Message Loop handles sending the Exit message to other loops."
        n114 = event-data() -> ()  [unwired: 1 in, 1 out]
        n115 = call-poly "Enqueue Message.vi"("Message Data"="StageY++" ("Message"), "Message"="StageControlChange", "Message Queue"=w247) -> ("error out"=w249:errorcluster, "dup Message Queue"=w246:refnum<queue>)  [unwired: 7 in]
      }
      event "StageZ-": Value Change {
        # "The UI Message Loop handles sending the Exit message to other loops."
        n116 = event-data() -> ()  [unwired: 1 in, 1 out]
        n117 = call-poly "Enqueue Message.vi"("Message Data"="StageZ-" ("Message"), "Message"="StageControlChange", "Message Queue"=w252) -> ("error out"=w254:errorcluster, "dup Message Queue"=w251:refnum<queue>)  [unwired: 7 in]
      }
      event "StageZ+": Value Change {
        # "The UI Message Loop handles sending the Exit message to other loops."
        n118 = event-data() -> ()  [unwired: 1 in, 1 out]
        n119 = call-poly "Enqueue Message.vi"("Message Data"="StageZ+" ("Message"), "Message"="StageControlChange", "Message Queue"=w257) -> ("error out"=w259:errorcluster, "dup Message Queue"=w256:refnum<queue>)  [unwired: 7 in]
      }
      event "StageZ--": Value Change {
        # "The UI Message Loop handles sending the Exit message to other loops."
        n120 = event-data() -> ()  [unwired: 1 in, 1 out]
        n121 = call-poly "Enqueue Message.vi"("Message Data"="StageZ--" ("Message"), "Message"="StageControlChange", "Message Queue"=w262) -> ("error out"=w264:errorcluster, "dup Message Queue"=w261:refnum<queue>)  [unwired: 7 in]
      }
      event "StageZ++": Value Change {
        # "The UI Message Loop handles sending the Exit message to other loops."
        n122 = event-data() -> ()  [unwired: 1 in, 1 out]
        n123 = call-poly "Enqueue Message.vi"("Message Data"="StageZ++" ("Message"), "Message"="StageControlChange", "Message Queue"=w267) -> ("error out"=w269:errorcluster, "dup Message Queue"=w266:refnum<queue>)  [unwired: 7 in]
      }
      event "TIRF-": Value Change {
        # "The UI Message Loop handles sending the Exit message to other loops."
        n124 = event-data() -> ()  [unwired: 1 in, 1 out]
        n125 = call-poly "Enqueue Message.vi"("Message Data"="TIRF-" ("Message"), "Message"="StageControlChange", "Message Queue"=w272) -> ("error out"=w274:errorcluster, "dup Message Queue"=w271:refnum<queue>)  [unwired: 7 in]
      }
      event "TIRF--": Value Change {
        # "The UI Message Loop handles sending the Exit message to other loops."
        n126 = event-data() -> ()  [unwired: 1 in, 1 out]
        n127 = call-poly "Enqueue Message.vi"("Message Data"="TIRF--" ("Message"), "Message"="StageControlChange", "Message Queue"=w277) -> ("error out"=w279:errorcluster, "dup Message Queue"=w276:refnum<queue>)  [unwired: 7 in]
      }
      event "EPI+": Value Change {
        # "The UI Message Loop handles sending the Exit message to other loops."
        n128 = event-data() -> ()  [unwired: 1 in, 1 out]
        n129 = call-poly "Enqueue Message.vi"("Message Data"="EPI+" ("Message"), "Message"="StageControlChange", "Message Queue"=w282) -> ("error out"=w284:errorcluster, "dup Message Queue"=w281:refnum<queue>)  [unwired: 7 in]
      }
      event "EPI++": Value Change {
        # "The UI Message Loop handles sending the Exit message to other loops."
        n130 = event-data() -> ()  [unwired: 1 in, 1 out]
        n131 = call-poly "Enqueue Message.vi"("Message Data"="EPI++" ("Message"), "Message"="StageControlChange", "Message Queue"=w287) -> ("error out"=w289:errorcluster, "dup Message Queue"=w286:refnum<queue>)  [unwired: 7 in]
      }
      event "TirfModuleScollBar": Value Change {
        # "The UI Message Loop handles sending the Exit message to other loops."
        n132 = event-data() -> ()  [unwired: 1 in, 1 out]
        n133 = call-poly "Enqueue Message.vi"("Message Data"="TirfModuleScollBarValueChange" ("Message"), "Message"="StageControlChange", "Message Queue"=w292) -> ("error out"=w294:errorcluster, "dup Message Queue"=w291:refnum<queue>)  [unwired: 7 in]
      }
      event "RawImage": Mouse Down {
        n134 = event-data() -> ("Coords"=w297:T16)  [unwired: 1 in, 4 out]
        n135 = Unbundle By Name(w297) -> ("Horizontal"=w296:i32, "Vertical"=w295:i32)
        n136 = global write "Global.vi" "MouseDownX"(w296) -> ()
        n137 = global write "Global.vi" "MouseDownY"(w295) -> ()
        n138 = global write "Global.vi" "MouseDownWithinImage"(TRUE ("MouseDownWithinImage")) -> ()
      }
      event "RawImage": Mouse Move {
        n139 = event-data() -> ("Coords"=w305:T16)  [unwired: 1 in, 4 out]
        n140 = global read "Global.vi" "MouseDownWithinImage"() -> (w300:bool)
        n141 = Unbundle By Name(w305) -> ("Horizontal"=w302:i32, "Vertical"=w301:i32)
        n142 = control-ref of="RawImage"() -> (w304:refnum<vi>)
        n143 = property on="Property Node" class="ImageControl"(reference=w304) -> ("Current ROI Tool"=w303:u32)  [unwired: 1 in, 2 out]
        n144 = call-poly "Enqueue Message.vi"("Message Data"="785" ("Message"), "Message"="Nop", "Message Queue"=w308) -> ("error out"=w310:errorcluster, "dup Message Queue"=w307:refnum<queue>)  [unwired: 7 in]
        n145 = case shown="True" w300 {
          tunnel: w303 -> [_ w313]
          tunnel: w302 -> [_ w312]
          tunnel: w301 -> [_ w311]
          frame False {
          }
          frame True {
            n146 = case shown="0..3" w313 {
              tunnel: w312 -> [_ _]
              tunnel: w311 -> [_ _]
              frame Default {
              }
              frame 0..3 {
              }
            }
          }
        }
      }
      event "RawImage": Mouse Wheel {
        n147 = event-data() -> ()  [unwired: 1 in, 10 out]
      }
      event "RawImage": Mouse Up {
        n148 = event-data() -> ()  [unwired: 1 in, 8 out]
        n149 = global write "Global.vi" "MouseDownWithinImage"(FALSE ("MouseDownWithinImage")) -> ()
      }
      event "RawImage": Drag Enter {
        w321 = TRUE  # Priority Message
        # "The UI Message Loop handles sending the Exit message to other loops."
        n150 = event-data() -> ()  [unwired: 1 in, 1 out]
        n151 = call-poly "Enqueue Message.vi"("Priority Message? (F)"=w321, "Message"="Exit", "Message Queue"=w320) -> ("error out"=w323:errorcluster, "dup Message Queue"=w319:refnum<queue>)  [unwired: 7 in]
        n152 = One Button Dialog(message="Drag", button name ("OK")="OK") -> ()  [unwired: 1 out]
        n153 = event-data() -> ()  [unwired: 2 in, 1 out]
      }
      event User Event {
        # "The Message Handling Loop processed an \"Exit\" message, which fired this event to stop the Event Handling Loop."
        n154 = event-data() -> ()  [unwired: 1 in, 1 out]
        n155 = local write "Status"("Exit" ("Exit String")) -> ()
      }
    }
    n156 = call "Error Handler - Event Handling Loop.vi"("error in (no error)"=w98, "Message Queue"=w97) -> ("dup error in"=w99:errorcluster)  [unwired: 8 in, 1 out]
  }
  n157 = call "Control Message Loop.vi"("error in (no error)"=w15, "DataQueuesAndNotifier"=w17, "Message Queues"=w22) -> ("error out"=w18:errorcluster)  [unwired: 8 in]
  n158 = call "Acquisition Message Loop.vi"("error in (no error)"=w15, "DataQueuesAndNotifier"=w17, "Message Queues"=w22) -> ("error out"=w19:errorcluster, "DataQueuesAndNotifier Out"=w21:T14)  [unwired: 7 in]
  n159 = while {
    tunnel: w23 -> [w339]
    tunnel: w38 -> [w344]
    shift-right: [w338] -> w14
    shift-left: "Config" -> [w337]
    shift-right: [w335] -> _
    shift-left: w43 -> [w336]
    tunnel: w26 -> [w334]
    tunnel: w25 -> [w333]
    shift-right: [w328] -> _
    shift-left: w42 -> [w329]
    tunnel: w37 -> [w343]
    tunnel: [w332] -> w48
    tunnel: w24 -> [w327]
    stop <- w345 stop-if-true
    # "UI Message Loop"
    n160 = call "Dequeue Message.vi"("error in (no error)"=w343, "Message Queue"=w339) -> ("error out"=w342:errorcluster, "Message Data"=w340:variant, "Message"=w341:string, "dup Message Queue"=w330:refnum<queue>)  [unwired: 6 in]
    n161 = case "Message Cases" shown="\"CameraSettingChange\"" w341 {
      selector: w341 -> [_ _ _ _ _ _ _ _ _ _ _ _ _ _ _ _ _ _ _ _ _ _ _ _ _ _ _ _ w965]
      tunnel: w330 -> [w350 w359 w393 w406 w418 _ w444 _ w466 w488 w489 w524 w550 w575 _ w615 w634 _ w648 _ _ _ _ _ _ _ _ _ _]
      tunnel: w342 -> [w351 w361 w395 w400 w420 w439 w448 w460 w469 w487 w499 w525 w551 w576 w608 w617 w628 w637 w647 w677 w696 w701 w709 w764 w776 w822 w947 w959 _]
      tunnel: [w346 w360 w394 w407 w422 w440 w454 w465 w469 w480 w500 w522 w548 w573 w605 w610 w631 w639 w646 w689 w695 w700 w715 w769 w783 w819 w950 w958 w964] -> w331
      tunnel: [_ _ _ _ _ _ _ _ _ _ _ _ _ _ _ _ _ _ _ TRUE _ _ _ _ _ _ _ _ _] -> w345
      tunnel: w340 -> [_ _ _ _ _ w438 _ _ _ _ _ _ _ _ _ _ _ w640 _ w679 _ _ w712 w766 w779 w824 _ w957 _]
      tunnel: w344 -> [_ _ _ _ _ _ _ _ _ _ _ _ _ _ _ _ _ _ _ w690 _ _ _ _ _ _ _ _ _]
      tunnel: [w348 w372 w385 w408 w413 w432 w443 w455 w471 w475 w496 w528 w554 w579 w599 w614 w625 w644 w651 w688 w694 w699 w710 w765 w777 w817 w948 w953 w968] -> w338
      tunnel: w337 -> [w354 w372 w385 w401 w413 w432 w443 w459 w471 w475 w496 w528 w554 w579 w599 w618 w626 w644 w651 w688 w694 w699 w710 w765 w777 w817 w948 w956 w968]
      tunnel: w336 -> [w353 w375 w397 w399 w414 w434 w442 w462 w470 w474 w495 w527 w553 w578 w600 w612 w633 w643 w650 w687 w693 w698 w702 w768 w782 w827 w952 w961 w967]
      tunnel: [w353 w365 w383 w399 w414 w434 w442 w462 w470 w474 w495 w527 w553 w578 w600 w612 w633 w643 w650 w687 w693 w698 w702 w768 w782 w827 w952 w961 w967] -> w335
      tunnel: w334 -> [_ _ _ w398 _ _ w453 w464 _ w479 w497 _ _ _ w602 _ _ _ _ w686 _ _ _ _ _ _ _ _ _]
      tunnel: w333 -> [_ _ _ _ _ _ _ _ _ w482 w498 _ _ _ w601 _ _ _ _ w685 _ _ _ _ _ _ _ _ _]
      tunnel: w329 -> [_ _ _ _ w421 w433 _ w461 w468 _ w491 w526 w552 w577 w609 w611 w632 w638 w649 _ w692 w697 w714 w767 w781 w826 w951 w963 w966]
      tunnel: [UI_State."Idle" ("UI State") UI_State."Idle" ("UI State") UI_State."Idle" ("UI State") UI_State."Idle" ("UI State") w421 w433 UI_State."Idle" ("UI State") w461 w468 UI_State."Acquiring and Logging" ("UI State") w490 w523 w549 w574 w609 w611 w632 w638 w645 UI_State."Idle" ("UI State") w692 w697 w714 w767 w781 w826 w951 w963 w966] -> w328
      tunnel: w327 -> [_ _ _ _ _ _ _ _ _ _ w492 _ _ _ w603 _ _ _ _ w674 _ _ w704 _ w770 w815 w946 _ _]
      frame "Initialize" {
        # "Load Setting"
        # "Initialize - Get configuration settings, Try to initialize and configrate the hardware, then message the UI to initialize, and broadcast the settings to the other message loops."
        n162 = call "Load Settings from XML.vi"("error in (no error)"=w351, "Settings in"=w354) -> ("error out"=w347:errorcluster, "Settings out"=w348:T2)  [unwired: 8 in]
        n163 = call-poly "Enqueue Message.vi"("error in (no error)"=w347, "Message"="Init UI Refs", "Message Queue"=w350) -> ("error out"=w346:errorcluster)  [unwired: 7 in, 1 out]
      }
      frame "Init UI Refs" {
        # "Init UI Refs - Store control references for UI controls.  Also enable/disable controls appropriately."
        n164 = control-ref of="Album"() -> (w374:refnum<vi>)
        n165 = control-ref of="Record"() -> (w371:refnum<vi>)
        n166 = control-ref of="Stop"() -> (w370:refnum<vi>)
        n167 = control-ref of="Settings"() -> (w369:refnum<vi>)
        n168 = control-ref of="Exit"() -> (w368:refnum<vi>)
        n169 = control-ref of="Status"() -> (w367:refnum<vi>)
        n170 = Bundle By Name(cluster=w375, "Album Ref"=w374, "Record Ref"=w371, "Stop Ref"=w370, "Settings Ref"=w369, "Exit Ref"=w368, "Status Ref"=w367) -> (w366:T12)
        n171 = control-ref of="405 nm"() -> (w364:refnum<vi>)
        n172 = control-ref of="488 nm"() -> (w363:refnum<vi>)
        n173 = control-ref of="532 nm"() -> (w362:refnum<vi>)
        n174 = control-ref of="561 nm"() -> (w357:refnum<vi>)
        n175 = control-ref of="647 nm"() -> (w356:refnum<vi>)
        n176 = control-ref of="785 nm"() -> (w355:refnum<vi>)
        n177 = Bundle By Name(cluster=w366, "405 Ref"=w364, "488 Ref"=w363, "532 Ref"=w362, "561 Ref"=w357, "647 Ref"=w356, "785 Ref"=w355) -> (w365:T12)
        n178 = call-poly "Enqueue Message.vi"("error in (no error)"=w361, "Message"="Init UI Refs1", "Message Queue"=w359) -> ("error out"=w360:errorcluster)  [unwired: 7 in, 1 out]
      }
      frame "Init UI Refs1" {
        # "Init UI Refs - Store control references for UI controls.  Also enable/disable controls appropriately."
        n179 = control-ref of="Power405"() -> (w391:refnum<vi>)
        n180 = control-ref of="Power488"() -> (w390:refnum<vi>)
        n181 = control-ref of="Power532"() -> (w389:refnum<vi>)
        n182 = control-ref of="Power561"() -> (w388:refnum<vi>)
        n183 = control-ref of="Power647"() -> (w387:refnum<vi>)
        n184 = control-ref of="Power785"() -> (w386:refnum<vi>)
        n185 = Bundle By Name(cluster=w397, "Power405 Ref"=w391, "Power488 Ref"=w390, "Power532 Ref"=w389, "Power561 Ref"=w388, "Power647 Ref"=w387, "Power785 Ref"=w386) -> (w384:T12)
        n186 = control-ref of="FrameIndexSroll"() -> (w377:refnum<vi>)
        n187 = control-ref of="CurrentFrame"() -> (w379:refnum<vi>)
        n188 = control-ref of="RealFPS"() -> (w378:refnum<vi>)
        n189 = control-ref of="DropFrame"() -> (w376:refnum<vi>)
        n190 = control-ref of="CapturingLED"() -> (w380:refnum<vi>)
        n191 = control-ref of="TIRF-Lock Z"() -> (w382:refnum<vi>)
        n192 = control-ref of="Anti-Drifft XY"() -> (w381:refnum<vi>)
        n193 = Bundle By Name(cluster=w384, "TIRFLock Ref"=w382, "AntiDrifft Ref"=w381, "Capturing"=w380, "FrameIndex"=w379, "RealFPS"=w378, "FrameIndexSroll"=w377, "DropFrame"=w376) -> (w383:T12)
        n194 = call-poly "Enqueue Message.vi"("error in (no error)"=w395, "Message"="Init And Config Devices", "Message Queue"=w393) -> ("error out"=w394:errorcluster)  [unwired: 7 in, 1 out]
      }
      frame "Init And Config Devices" {
        # "Config Devices"
        # "Initialize Devices"
        # "Load Setting"
        # "Initialize - Get configuration settings, Try to initialize and configrate the hardware, then message the UI to initialize, and broadcast the settings to the other message loops."
        n195 = call "Initialize Hardware References.vi"("error in (no error)"=w400, "Config In"=w401) -> ("error out"=w410:errorcluster, "Config Out"=w409:T2)  [unwired: 4 in]
        n196 = call "Configure Hardware.vi"("error in (no error)"=w410, "Acquisition"=w398, "UI Refs"=w399, "Config In"=w409) -> ("error out"=w403:errorcluster, "Config Out"=w408:T2)  [unwired: 6 in]
        n197 = call-poly "Enqueue Message.vi"("error in (no error)"=w403, "Message"="Broadcast Settings", "Message Queue"=w406) -> ("error out"=w404:errorcluster, "dup Message Queue"=w405:refnum<queue>)  [unwired: 7 in]
        n198 = call-poly "Enqueue Message.vi"("error in (no error)"=w404, "Message"="Init Finish", "Message Queue"=w405) -> ("error out"=w407:errorcluster)  [unwired: 7 in, 1 out]
      }
      frame "Init Finish" {
        # "Duplicate this frame when creating new messages.  Change this comment in the duplicated frame to describe this message."
        n199 = Unbundle By Name(w413) -> ("HardWare Status.CameraAndStages"=w416:T7, "HardWare Status.CameraAndStages.Camera"=w417:bool)
        n200 = case shown="True" w417 {
          tunnel: w420 -> [w427 w431]
          tunnel: [w426 w430] -> w419
          tunnel: w418 -> [w423 w429]
          frame False {
            n201 = call-poly "Enqueue Message.vi"("error in (no error)"=w427, "Message Data"="Preview..." ("Acquiring and Logging..."), "Message"="Update Status", "Message Queue"=w423) -> ("error out"=w426:errorcluster)  [unwired: 6 in, 1 out]
          }
          frame True {
            n202 = call-poly "Enqueue Message.vi"("error in (no error)"=w431, "Message"="Live", "Message Queue"=w429) -> ("error out"=w430:errorcluster)  [unwired: 7 in, 1 out]
          }
        }
        n203 = local write "DeviceStatus"(w416) -> ()
        n204 = Merge Errors(w419) -> (w422:errorcluster)
        n205 = call "Set All Controls Status.vi"("String"="Init", "UI Refs"=w414, "Config"=w413) -> ()  [unwired: 9 in]
      }
      frame "Update Status" {
        # "Update Status - Convert the message data to a string to display in the Status indicator."
        n206 = Variant To Data(error in=w439, type="", Variant=w438) -> (data=→"Status":string, error out=w436:errorcluster)
        n207 = Merge Errors "Merge Errors"(w436) -> (w440:errorcluster)
      }
      frame "Live" {
        # "Message Acquisition loops to start."
        # "Start - Enable/Disable buttons appropriately for an acquisition that has started, and update status display."
        n208 = local write "RecordLED"(FALSE ("RecordLED")) -> ()
        n209 = local write "LiveLED"(TRUE ("RecordLED")) -> ()
        n210 = call-poly "Enqueue Message.vi"("error in (no error)"=w448, "Message Data"="Preview..." ("Acquiring and Logging..."), "Message"="Update Status", "Message Queue"=w444) -> ("error out"=w447:errorcluster)  [unwired: 6 in, 1 out]
        n211 = call "Set All Controls Status.vi"("String"="Live", "UI Refs"=w442, "Config"=w443) -> ()  [unwired: 9 in]
        n212 = call-poly "Enqueue Message.vi"("error in (no error)"=w447, "Message"="Live", "Message Queue"=w453) -> ("error out"=w454:errorcluster)  [unwired: 7 in, 1 out]
      }
      frame "CameraSettingChange" {
        # "Start - Enable/Disable buttons appropriately for an acquisition that has started, and update status display."
        n213 = Bundle By Name(cluster=w459, "Hardware Configuration.Camera Configuration.Setting.Expouse"="Exposure", "Hardware Configuration.Camera Configuration.Setting.Frames"="CaptureFrame", "Hardware Configuration.Camera Configuration.Setting.FrameRate"="FrameRate") -> (w455:T2)
        n214 = call-poly "Enqueue Message.vi"("error in (no error)"=w460, "Message Data"=w455, "Message"="CameraSettingChange", "Message Queue"=w464) -> ("error out"=w465:errorcluster)  [unwired: 6 in, 1 out]
      }
      frame "Album" {
        # "Start - Enable/Disable buttons appropriately for an acquisition that has started, and update status display."
        n215 = call-poly "Enqueue Message.vi"("Message"="Live", "Message Queue"=w466) -> ()  [unwired: 8 in, 2 out]
      }
      frame "Record" {
        # "Message Acquisition and Logging loops to start."
        # "Start - Enable/Disable buttons appropriately for an acquisition that has started, and update status display."
        n216 = local write "RecordLED"(TRUE ("RecordLED")) -> ()
        n217 = local write "LiveLED"(FALSE ("RecordLED")) -> ()
        n218 = call-poly "Enqueue Message.vi"("error in (no error)"=w487, "Message Data"="Recording and logging" ("Acquiring and Logging..."), "Message"="Update Status", "Message Queue"=w488) -> ("error out"=w484:errorcluster)  [unwired: 6 in, 1 out]
        n219 = call-poly "Enqueue Message.vi"("error in (no error)"=w484, "Message"="Start", "Message Queue"=w482) -> ("error out"=w481:errorcluster)  [unwired: 7 in, 1 out]
        n220 = call "Set All Controls Status.vi"("String"="Record", "UI Refs"=w474, "Config"=w475) -> ()  [unwired: 9 in]
        n221 = call-poly "Enqueue Message.vi"("error in (no error)"=w481, "Message"="Record", "Message Queue"=w479) -> ("error out"=w480:errorcluster)  [unwired: 7 in, 1 out]
      }
      frame "Stop" {
        # "Stop - Enable/Disable buttons appropriately for an acquisition that has stopped, and update status display."
        n222 = case shown="\"Acquiring and Logging\"" w491 {
          selector: w491 -> [w501 w510 _]
          tunnel: w499 -> [w509 w511 w521]
          tunnel: w498 -> [w508 _ w520]
          tunnel: w497 -> [w506 _ w518]
          tunnel: [w504 w511 w514] -> w493
          tunnel: w492 -> [w503 _ _]
          tunnel: [w501 w510 UI_State."Idle" ("UI State")] -> w490
          tunnel: w489 -> [_ _ w513]
          frame "Waiting for Exit" {
            w502 = "Stop" ("Message")
            n223 = call-poly "Enqueue Message.vi"("error in (no error)"=w509, "Message"=w502, "Message Queue"=w508) -> ("error out"=w507:errorcluster)  [unwired: 7 in, 1 out]
            n224 = call-poly "Enqueue Message.vi"("error in (no error)"=w507, "Message"=w502, "Message Queue"=w506) -> ("error out"=w505:errorcluster)  [unwired: 7 in, 1 out]
            n225 = call-poly "Enqueue Message.vi"("error in (no error)"=w505, "Message"=w502, "Message Queue"=w503) -> ("error out"=w504:errorcluster)  [unwired: 7 in, 1 out]
          }
          frame Default {
          }
          frame "Acquiring and Logging" {
            w517 = "Stop" ("Message")
            n226 = call-poly "Enqueue Message.vi"("error in (no error)"=w521, "Message"=w517, "Message Queue"=w520) -> ("error out"=w519:errorcluster)  [unwired: 7 in, 1 out]
            n227 = call-poly "Enqueue Message.vi"("error in (no error)"=w519, "Message"=w517, "Message Queue"=w518) -> ("error out"=w515:errorcluster)  [unwired: 7 in, 1 out]
            n228 = call-poly "Enqueue Message.vi"("error in (no error)"=w515, "Message"="Live", "Message Queue"=w513) -> ("error out"=w514:errorcluster)  [unwired: 7 in, 1 out]
          }
        }
        n229 = call "Set All Controls Status.vi"("String"="Stop", "UI Refs"=w495, "Config"=w496) -> ()  [unwired: 9 in]
        n230 = Merge Errors(w493) -> (w500:errorcluster)
      }
      frame "Acquisition Stopped" {
        # "Logic for determining what action to take when the acquisition has stopped."
        n231 = case shown="\"Waiting for Exit\", \"Waiting for Exit (Acq Stopped)\"" w526 {
          selector: w526 -> [w530 _ _ _ _]
          tunnel: w525 -> [w529 w532 w534 w541 w547]
          tunnel: w524 -> [_ _ _ w539 w544]
          tunnel: [w530 UI_State."Waiting for Exit (Acq Stopped)" ("UI State") UI_State."Waiting for Stop (Acq Stopped)" ("UI State") UI_State."Idle" ("UI State") UI_State."Idle" ("UI State")] -> w523
          tunnel: [w529 w532 w534 w540 w545] -> w522
          frame Default {
            # "The initial state is waiting for stop(5), It is a default state .\nBecouse logging stop will alway comes later than acquisition stop msg"
          }
          frame "Waiting for Exit", "Waiting for Exit (Acq Stopped)" {
          }
          frame "Waiting for Stop", "Waiting for Stop (Acq Stopped)" {
          }
          frame "Waiting for Exit (Log Stopped)" {
            # "If we are waiting to exit, and the logging has already stopped, then the \"Acquisition Stopped\" message indicates that it is time to exit."
            n232 = call-poly "Enqueue Message.vi"("Priority Message? (F)"=TRUE, "error in (no error)"=w541, "Message"="Exit", "Message Queue"=w539) -> ("error out"=w540:errorcluster)  [unwired: 6 in, 1 out]
            n233 = Wait (ms)(milliseconds to wait=u32 100) -> ()  [unwired: 1 out]
          }
          frame "Waiting for Stop (Log Stopped)" {
            # "If we are waiting to stop, and the logging has already stopped, then the \"Acquisition Stopped\" message indicates that it is time to stop."
            n234 = call-poly "Enqueue Message.vi"("error in (no error)"=w547, "Message Data"="Ready..." ("Ready..."), "Message"="Update Status", "Message Queue"=w544) -> ("error out"=w545:errorcluster)  [unwired: 6 in, 1 out]
          }
        }
      }
      frame "Control Stopped" {
        # "Logic for determining what action to take when the acquisition has stopped."
        n235 = case shown="\"Waiting for Stop (Log Stopped)\"" w552 {
          selector: w552 -> [w556 _ _ _ _]
          tunnel: w551 -> [w555 w558 w560 w566 w572]
          tunnel: w550 -> [_ _ _ w564 w569]
          tunnel: [w556 UI_State."Waiting for Exit (Acq Stopped)" ("UI State") UI_State."Waiting for Stop (Acq Stopped)" ("UI State") UI_State."Idle" ("UI State") UI_State."Idle" ("UI State")] -> w549
          tunnel: [w555 w558 w560 w565 w570] -> w548
          frame Default {
            # "The initial state is waiting for stop(5), It is a default state .\nBecouse logging stop will alway comes later than acquisition stop msg"
          }
          frame "Waiting for Exit", "Waiting for Exit (Acq Stopped)" {
          }
          frame "Waiting for Stop", "Waiting for Stop (Acq Stopped)" {
          }
          frame "Waiting for Exit (Log Stopped)" {
            # "If we are waiting to exit, and the logging has already stopped, then the \"Acquisition Stopped\" message indicates that it is time to exit."
            n236 = call-poly "Enqueue Message.vi"("Priority Message? (F)"=TRUE, "error in (no error)"=w566, "Message"="Exit", "Message Queue"=w564) -> ("error out"=w565:errorcluster)  [unwired: 6 in, 1 out]
          }
          frame "Waiting for Stop (Log Stopped)" {
            # "If we are waiting to stop, and the logging has already stopped, then the \"Acquisition Stopped\" message indicates that it is time to stop."
            n237 = call-poly "Enqueue Message.vi"("error in (no error)"=w572, "Message Data"="Ready..." ("Ready..."), "Message"="Update Status", "Message Queue"=w569) -> ("error out"=w570:errorcluster)  [unwired: 6 in, 1 out]
          }
        }
      }
      frame "Logging Stopped" {
        # "Logic for determining what action to take when the logging has stopped."
        n238 = case shown="\"Waiting for Stop\", \"Waiting for Stop (Log Stopped)\"" w577 {
          selector: w577 -> [w581 _ _ _ _]
          tunnel: w576 -> [w580 w583 w585 w592 w595]
          tunnel: w575 -> [_ _ _ w590 w594]
          tunnel: [w581 UI_State."Waiting for Exit (Log Stopped)" ("UI State") UI_State."Waiting for Stop (Log Stopped)" ("UI State") UI_State."Idle" ("UI State") UI_State."Idle" ("UI State")] -> w574
          tunnel: [w580 w583 w585 w591 w593] -> w573
          frame Default {
          }
          frame "Waiting for Exit", "Waiting for Exit (Log Stopped)" {
          }
          frame "Waiting for Stop", "Waiting for Stop (Log Stopped)" {
          }
          frame "Waiting for Exit (Acq Stopped)" {
            # "If we are waiting to exit, and the acquisition has already stopped, then the \"Logging Stopped\" message indicates that it is time to exit."
            n239 = call-poly "Enqueue Message.vi"("Priority Message? (F)"=TRUE, "error in (no error)"=w592, "Message"="Exit", "Message Queue"=w590) -> ("error out"=w591:errorcluster)  [unwired: 6 in, 1 out]
            n240 = Wait (ms)(milliseconds to wait=u32 100) -> ()  [unwired: 1 out]
          }
          frame "Waiting for Stop (Acq Stopped)" {
            # "If we are waiting to stop, and the acquisition has already stopped, then the \"Logging Stopped\" message indicates that it is time to stop."
            n241 = call-poly "Enqueue Message.vi"("error in (no error)"=w595, "Message Data"="Ready..." ("Ready..."), "Message"="Update Status", "Message Queue"=w594) -> ("error out"=w593:errorcluster)  [unwired: 6 in, 1 out]
          }
        }
      }
      frame "Broadcast settings" {
        w604 = "Update Settings" ("Message")
        # "Broadcast settings - Send the 'Update Settings' message to the Logging and Acquisition message loops."
        n242 = call-poly "Enqueue Message.vi"("error in (no error)"=w608, "Message Data"=w599, "Message"=w604, "Message Queue"=w601) -> ("error out"=w607:errorcluster)  [unwired: 6 in, 1 out]
        n243 = call-poly "Enqueue Message.vi"("error in (no error)"=w607, "Message Data"=w599, "Message"=w604, "Message Queue"=w602) -> ("error out"=w606:errorcluster)  [unwired: 6 in, 1 out]
        n244 = call-poly "Enqueue Message.vi"("error in (no error)"=w606, "Message Data"=w599, "Message"=w604, "Message Queue"=w603) -> ("error out"=w605:errorcluster)  [unwired: 6 in, 1 out]
      }
      frame "Launch Settings Dialog" {
        # "Launch Settings Dialog - Launch the Settings Dialog when the user clicks the 'Settings' button."
        n245 = call-by-ref "?"("error in (no error)"=w617, "Settings in"=w618) -> ("error out"=w613:errorcluster, "Cancelled?"=w616:bool, "Settings out"=w614:T2)  [unwired: 8 in, 3 out]
        n246 = case shown="False" w616 {
          tunnel: w615 -> [w622 _]
          tunnel: w613 -> [w621 w623]
          tunnel: [w620 w623] -> w610
          frame False {
            n247 = call-poly "Enqueue Message.vi"("error in (no error)"=w621, "Message"="Broadcast Settings", "Message Queue"=w622) -> ("error out"=w620:errorcluster)  [unwired: 7 in, 1 out]
          }
          frame True {
          }
        }
      }
      frame "Save Settings" {
        # "Launch Settings Dialog - Launch the Settings Dialog when the user clicks the 'Settings' button."
        n248 = call "Save Settings to XML.vi"("error in (no error)"=w628, "SaveDefault=false"=TRUE, "Settings"=w626) -> ("error out"=w627:errorcluster, "Settings Out"=w625:T2)  [unwired: 7 in]
        n249 = call-poly "Enqueue Message.vi"("error in (no error)"=w627, "Message Data"="Setting configuration saved" ("Message"), "Message"="Update Status", "Message Queue"=w634) -> ("error out"=w631:errorcluster)  [unwired: 6 in, 1 out]
      }
      frame "Error" {
        # "Error - Display an error dialog. This message is sent by the \"Error Handler\" VIs at the end of other loops in this application."
        n250 = Variant To Data(error in=w637, type=errorcluster {"status"=FALSE, "code"=0, "source"=""} ("error constant"), Variant=w640) -> (data=w636:errorcluster, error out=w641:errorcluster)
        n251 = Unbundle By Name(w636) -> ("source"=w635:string)
        n252 = local write "Status"(w635) -> ()
        n253 = Merge Errors(w641) -> (w639:errorcluster)
      }
      frame "Confirm Quit" {
        # "Confirm Quit - Message that can confirm whether or not the user wants to exit the application."
        n254 = case shown="\"Acquiring and Logging\"" w649 {
          tunnel: w648 -> [w658 w662]
          tunnel: w647 -> [w657 w661]
          tunnel: [w656 w660] -> w646
          tunnel: [UI_State."Waiting for Exit" ("UI State") w659] -> w645
          frame Default {
            # "If 'Confirm Quit' comes in while the system is idle, there is no need for a confirmation message."
            n255 = call-poly "Enqueue Message.vi"("Priority Message? (F)"=TRUE, "error in (no error)"=w657, "Message"="Stop", "Message Queue"=w658) -> ("error out"=w656:errorcluster)  [unwired: 6 in, 1 out]
            n256 = Wait (ms)(milliseconds to wait=u32 100) -> ()  [unwired: 1 out]
          }
          frame "Acquiring and Logging" {
            n257 = Two Button Dialog(message="Are you sure you want to quit while the acquisition is running?" ("Confirm Quit Message"), 1:"No" ("No"), 2:"Yes" ("Yes")) -> (T button?=w663:bool)
            n258 = case shown="True" w663 {
              tunnel: w662 -> [_ w672]
              tunnel: w661 -> [w668 w673]
              tunnel: [w668 w671] -> w660
              tunnel: [UI_State."Acquiring and Logging" ("UI State") UI_State."Waiting for Exit" ("UI State")] -> w659
              frame False {
                # "User did not want to quit."
              }
              frame True {
                n259 = call-poly "Enqueue Message.vi"("error in (no error)"=w673, "Message"="Stop", "Message Queue"=w672) -> ("error out"=w671:errorcluster)  [unwired: 7 in, 1 out]
              }
            }
          }
        }
      }
      frame "Exit" {
        w682 = TRUE ("Priority Message? (F)")
        w675 = "Exit" ("Message")
        # "Popup an error dialog if 'Exit' was called as a result of an error."
        # "Stop the VI"
        # "Exit - Send Exit messages to the Acquisition and Logging loops, and fire the user event to stop the Event Handling Loop."
        n260 = Variant To Data(type=errorcluster {"status"=FALSE, "code"=0, "source"=""} ("error constant"), Variant=w679) -> (data=w678:errorcluster)  [unwired: 1 in, 1 out]
        n261 = call-poly "Enqueue Message.vi"("error in (no error)"=w677, "Message"=w675, "Message Queue"=w674) -> ("error out"=w676:errorcluster)  [unwired: 7 in, 1 out]
        n262 = call <vilib>:"Simple Error Handler.vi"("error in (no error)"=w678) -> ()  [unwired: 4 in, 5 out]
        n263 = call-poly "Enqueue Message.vi"("Priority Message? (F)"=w682, "error in (no error)"=w676, "Message"=w675, "Message Queue"=w686) -> ("error out"=w683:errorcluster)  [unwired: 6 in, 1 out]
        n264 = call-poly "Enqueue Message.vi"("Priority Message? (F)"=w682, "error in (no error)"=w683, "Message"=w675, "Message Queue"=w685) -> ("error out"=w681:errorcluster)  [unwired: 6 in, 1 out]
        n265 = call "Fire User Event - Stop.vi"("error in (no error)"=w681, "User Event - Stop"=w690) -> ("error out"=w689:errorcluster)  [unwired: 9 in]
      }
      frame "---Copy This Frame---" {
        # "Duplicate this frame when creating new messages.  Change this comment in the duplicated frame to describe this message."
        n266 = Merge Errors(w696) -> (w695:errorcluster)
      }
      frame "Nop" {
        # "Duplicate this frame when creating new messages.  Change this comment in the duplicated frame to describe this message."
        n267 = Merge Errors(w701) -> (w700:errorcluster)
      }
      frame "LasersSwitch" {
        # "Duplicate this frame when creating new messages.  Change this comment in the duplicated frame to describe this message."
        n268 = Variant To Data(error in=w709, type="", Variant=w712) -> (data=w711:string, error out=w705:errorcluster)
        n269 = case shown="\"647\"" w711 {
          tunnel: w710 -> [_ w723 w730 w737 w744 w751 w758]
          tunnel: T17 {"Laser Ref"=refnum, "statue"=FALSE, "Power"=0.0, "Power Ref"=refnum} ("Laser Ctrl") -> [w716 w721 w729 w736 w743 w750 w757]
          tunnel: [w716 w722 w728 w735 w742 w749 w756] -> w703
          tunnel: w702 -> [_ w718 w725 w732 w738 w745 w752]
          frame Default {
          }
          frame "405" {
            n270 = Unbundle By Name(w718) -> ("Power405 Ref"=w717:refnum<vi>)
            n271 = local read "405 nm"() -> (w720:bool)
            n272 = Unbundle By Name(w723) -> ("Hardware Configuration.Lasers Configuration.Resource.Lasers Ref.405 Ref"=w719:refnum<k24>)
            n273 = Bundle By Name(cluster=w721, "Laser Ref"=w719, "Power Ref"=w717, "statue"=w720) -> (w722:T17)
          }
          frame "488" {
            n274 = Unbundle By Name(w725) -> ("Power488 Ref"=w724:refnum<vi>)
            n275 = local read "488 nm"() -> (w727:bool)
            n276 = Unbundle By Name(w730) -> ("Hardware Configuration.Lasers Configuration.Resource.Lasers Ref.488 Ref"=w726:refnum<k24>)
            n277 = Bundle By Name(cluster=w729, "Laser Ref"=w726, "Power Ref"=w724, "statue"=w727) -> (w728:T17)
          }
          frame "532" {
            n278 = Unbundle By Name(w732) -> ("Power532 Ref"=w733:refnum<vi>)
            n279 = local read "532 nm"() -> (w731:bool)
            n280 = Unbundle By Name(w737) -> ("Hardware Configuration.Lasers Configuration.Resource.Lasers Ref.532 Ref"=w734:refnum<k24>)
            n281 = Bundle By Name(cluster=w736, "Laser Ref"=w734, "Power Ref"=w733, "statue"=w731) -> (w735:T17)
          }
          frame "561" {
            n282 = Unbundle By Name(w738) -> ("Power561 Ref"=w739:refnum<vi>)
            n283 = local read "561 nm"() -> (w741:bool)
            n284 = Unbundle By Name(w744) -> ("Hardware Configuration.Lasers Configuration.Resource.Lasers Ref.561 Ref"=w740:refnum<k24>)
            n285 = Bundle By Name(cluster=w743, "Laser Ref"=w740, "Power Ref"=w739, "statue"=w741) -> (w742:T17)
          }
          frame "647" {
            n286 = Unbundle By Name(w745) -> ("Power647 Ref"=w746:refnum<vi>)
            n287 = local read "647 nm"() -> (w748:bool)
            n288 = Unbundle By Name(w751) -> ("Hardware Configuration.Lasers Configuration.Resource.Lasers Ref.647 Ref"=w747:refnum<k24>)
            n289 = Bundle By Name(cluster=w750, "Laser Ref"=w747, "Power Ref"=w746, "statue"=w748) -> (w749:T17)
          }
          frame "785" {
            n290 = Unbundle By Name(w752) -> ("Power785 Ref"=w753:refnum<vi>)
            n291 = local read "785 nm"() -> (w754:bool)
            n292 = Unbundle By Name(w758) -> ("Hardware Configuration.Lasers Configuration.Resource.Lasers Ref.785 Ref"=w755:refnum<k24>)
            n293 = Bundle By Name(cluster=w757, "Laser Ref"=w755, "Power Ref"=w753, "statue"=w754) -> (w756:T17)
          }
        }
        n294 = call-poly "Enqueue Message.vi"("error in (no error)"=w705, "Message Data"=w703, "Message"="LasersSwitch", "Message Queue"=w704) -> ("error out"=w708:errorcluster)  [unwired: 6 in, 1 out]
        n295 = Merge Errors(w708) -> (w715:errorcluster)
      }
      frame "UpdateLaserPower" {
        # "Duplicate this frame when creating new messages.  Change this comment in the duplicated frame to describe this message."
        n296 = Variant To Data(error in=w764, type=T17 {"Laser Ref"=refnum, "statue"=FALSE, "Power"=0.0, "Power Ref"=refnum} ("Laser Ctrl"), Variant=w766) -> (data=w761:T17, error out=w762:errorcluster)
        n297 = Unbundle By Name(w761) -> ("Power Ref"=w760:refnum<vi>, "Power"=w759:dbl)
        n298 = property class="DigNum"(reference=w760, "Value"=w759) -> ()  [unwired: 1 in, 2 out]
        n299 = Merge Errors(w762) -> (w769:errorcluster)
      }
      frame "LasersPowerChange" {
        # "Duplicate this frame when creating new messages.  Change this comment in the duplicated frame to describe this message."
        n300 = Variant To Data(error in=w776, type="", Variant=w779) -> (data=w778:string, error out=w771:errorcluster)
        n301 = case shown="\"785\"" w778 {
          tunnel: w777 -> [_ w789 w794 w799 w804 w809 w814]
          tunnel: T17 {"Laser Ref"=refnum, "statue"=FALSE, "Power"=0.0, "Power Ref"=refnum} ("Laser Ctrl") -> [w784 w787 w793 w798 w803 w808 w813]
          tunnel: [w784 w788 w792 w797 w802 w807 w812] -> w772
          frame Default {
          }
          frame "405" {
            n302 = local read "Power405"() -> (w786:dbl)
            n303 = Unbundle By Name(w789) -> ("Hardware Configuration.Lasers Configuration.Resource.Lasers Ref.405 Ref"=w785:refnum<k24>)
            n304 = Bundle By Name(cluster=w787, "Laser Ref"=w785, "Power"=w786) -> (w788:T17)
          }
          frame "488" {
            n305 = local read "Power488"() -> (w791:dbl)
            n306 = Unbundle By Name(w794) -> ("Hardware Configuration.Lasers Configuration.Resource.Lasers Ref.488 Ref"=w790:refnum<k24>)
            n307 = Bundle By Name(cluster=w793, "Laser Ref"=w790, "Power"=w791) -> (w792:T17)
          }
          frame "532" {
            n308 = local read "Power532"() -> (w796:sgl)
            n309 = Unbundle By Name(w799) -> ("Hardware Configuration.Lasers Configuration.Resource.Lasers Ref.532 Ref"=w795:refnum<k24>)
            n310 = Bundle By Name(cluster=w798, "Laser Ref"=w795, "Power"=w796) -> (w797:T17)
          }
          frame "561" {
            n311 = local read "Power561"() -> (w801:dbl)
            n312 = Unbundle By Name(w804) -> ("Hardware Configuration.Lasers Configuration.Resource.Lasers Ref.561 Ref"=w800:refnum<k24>)
            n313 = Bundle By Name(cluster=w803, "Laser Ref"=w800, "Power"=w801) -> (w802:T17)
          }
          frame "647" {
            n314 = local read "Power647"() -> (w806:sgl)
            n315 = Unbundle By Name(w809) -> ("Hardware Configuration.Lasers Configuration.Resource.Lasers Ref.647 Ref"=w805:refnum<k24>)
            n316 = Bundle By Name(cluster=w808, "Laser Ref"=w805, "Power"=w806) -> (w807:T17)
          }
          frame "785" {
            n317 = local read "Power785"() -> (w810:dbl)
            n318 = Unbundle By Name(w814) -> ("Hardware Configuration.Lasers Configuration.Resource.Lasers Ref.785 Ref"=w811:refnum<k24>)
            n319 = Bundle By Name(cluster=w813, "Laser Ref"=w811, "Power"=w810) -> (w812:T17)
          }
        }
        n320 = call-poly "Enqueue Message.vi"("error in (no error)"=w771, "Message Data"=w772, "Message"="LasersPowerChange", "Message Queue"=w770) -> ("error out"=w775:errorcluster)  [unwired: 6 in, 1 out]
        n321 = Merge Errors(w775) -> (w783:errorcluster)
      }
      frame "StageControlChange" {
        # "Duplicate this frame when creating new messages.  Change this comment in the duplicated frame to describe this message."
        n322 = Variant To Data(error in=w822, type="", Variant=w824) -> (data=w823:string, error out=w821:errorcluster)
        n323 = case shown="\"EPI+\"" w823 {
          tunnel: w821 -> [w829 w836 w843 w850 w857 w864 w871 w878 w885 w892 w899 w906 w913 w919 w927 w935 w943]
          tunnel: [w829 w835 w842 w849 w856 w863 w870 w877 w884 w891 w898 w905 w912 w918 w926 w934 w942] -> w820
          tunnel: [T18 {"Axis"=0.0, "value"=0.0, "direction"=FALSE} ("Stage Ctrl") w830 w837 w844 w851 w858 w865 w872 w879 w886 w893 w900 w907 w914 w923 w931 w939] -> w816
          frame Default {
          }
          frame "StageX-" {
            n324 = local read "XYIncreatement+"() -> (w833:dbl)
            n325 = Multiply(x=-1.0, y=w833) -> (x*y=w832:dbl)
            n326 = call "Package stage data to cluster.vi"("error in (no error)"=w836, "Increasement"=w832, "axis"=u32 1) -> ("error out"=w835:errorcluster, "Stage Ctrl"=w830:T18)  [unwired: 6 in]
          }
          frame "StageX+" {
            n327 = local read "XYIncreatement+"() -> (w840:dbl)
            n328 = Multiply(x=1.0, y=w840) -> (x*y=w839:dbl)
            n329 = call "Package stage data to cluster.vi"("error in (no error)"=w843, "Increasement"=w839, "axis"=u32 1) -> ("error out"=w842:errorcluster, "Stage Ctrl"=w837:T18)  [unwired: 6 in]
          }
          frame "StageY-" {
            n330 = local read "XYIncreatement+"() -> (w847:dbl)
            n331 = Multiply(x=-1.0, y=w847) -> (x*y=w846:dbl)
            n332 = call "Package stage data to cluster.vi"("error in (no error)"=w850, "Increasement"=w846, "axis"=u32 2) -> ("error out"=w849:errorcluster, "Stage Ctrl"=w844:T18)  [unwired: 6 in]
          }
          frame "StageY+" {
            n333 = local read "XYIncreatement+"() -> (w854:dbl)
            n334 = Multiply(x=1.0, y=w854) -> (x*y=w853:dbl)
            n335 = call "Package stage data to cluster.vi"("error in (no error)"=w857, "Increasement"=w853, "axis"=u32 2) -> ("error out"=w856:errorcluster, "Stage Ctrl"=w851:T18)  [unwired: 6 in]
          }
          frame "StageX--" {
            n336 = local read "XYIncreatement++"() -> (w861:dbl)
            n337 = Multiply(x=-1.0, y=w861) -> (x*y=w860:dbl)
            n338 = call "Package stage data to cluster.vi"("error in (no error)"=w864, "Increasement"=w860, "axis"=u32 1) -> ("error out"=w863:errorcluster, "Stage Ctrl"=w858:T18)  [unwired: 6 in]
          }
          frame "StageX++" {
            n339 = local read "XYIncreatement++"() -> (w868:dbl)
            n340 = Multiply(x=1.0, y=w868) -> (x*y=w867:dbl)
            n341 = call "Package stage data to cluster.vi"("error in (no error)"=w871, "Increasement"=w867, "axis"=u32 1) -> ("error out"=w870:errorcluster, "Stage Ctrl"=w865:T18)  [unwired: 6 in]
          }
          frame "StageY++" {
            n342 = local read "XYIncreatement++"() -> (w875:dbl)
            n343 = Multiply(x=1.0, y=w875) -> (x*y=w874:dbl)
            n344 = call "Package stage data to cluster.vi"("error in (no error)"=w878, "Increasement"=w874, "axis"=u32 2) -> ("error out"=w877:errorcluster, "Stage Ctrl"=w872:T18)  [unwired: 6 in]
          }
          frame "StageY--" {
            n345 = local read "XYIncreatement++"() -> (w882:dbl)
            n346 = Multiply(x=-1.0, y=w882) -> (x*y=w881:dbl)
            n347 = call "Package stage data to cluster.vi"("error in (no error)"=w885, "Increasement"=w881, "axis"=u32 2) -> ("error out"=w884:errorcluster, "Stage Ctrl"=w879:T18)  [unwired: 6 in]
          }
          frame "StageZ-" {
            n348 = local read "ZIncreatement+"() -> (w889:dbl)
            n349 = Multiply(x=-1.0, y=w889) -> (x*y=w888:dbl)
            n350 = call "Package stage data to cluster.vi"("error in (no error)"=w892, "Increasement"=w888, "axis"=u32 3) -> ("error out"=w891:errorcluster, "Stage Ctrl"=w886:T18)  [unwired: 6 in]
          }
          frame "StageZ+" {
            n351 = local read "ZIncreatement+"() -> (w896:dbl)
            n352 = Multiply(x=1.0, y=w896) -> (x*y=w895:dbl)
            n353 = call "Package stage data to cluster.vi"("error in (no error)"=w899, "Increasement"=w895, "axis"=u32 3) -> ("error out"=w898:errorcluster, "Stage Ctrl"=w893:T18)  [unwired: 6 in]
          }
          frame "StageZ--" {
            n354 = local read "ZIncreatement++"() -> (w903:dbl)
            n355 = Multiply(x=-1.0, y=w903) -> (x*y=w902:dbl)
            n356 = call "Package stage data to cluster.vi"("error in (no error)"=w906, "Increasement"=w902, "axis"=u32 3) -> ("error out"=w905:errorcluster, "Stage Ctrl"=w900:T18)  [unwired: 6 in]
          }
          frame "StageZ++" {
            n357 = local read "ZIncreatement++"() -> (w910:dbl)
            n358 = Multiply(x=1.0, y=w910) -> (x*y=w909:dbl)
            n359 = call "Package stage data to cluster.vi"("error in (no error)"=w913, "Increasement"=w909, "axis"=u32 3) -> ("error out"=w912:errorcluster, "Stage Ctrl"=w907:T18)  [unwired: 6 in]
          }
          frame "TIRF-" {
            n360 = local read "MicroStage+"() -> (w920:dbl)
            n361 = Multiply(x=1.0, y=w920) -> (x*y=w917:dbl)
            n362 = call "Package stage data to cluster.vi"("error in (no error)"=w919, "Increasement"=w917, "axis"=u32 4, "direction"=FALSE ("Direction")) -> ("error out"=w918:errorcluster, "Stage Ctrl"=w914:T18)  [unwired: 5 in]
          }
          frame "TIRF--" {
            n363 = local read "MicroStage+"() -> (w928:dbl)
            n364 = Multiply(x=10.0, y=w928) -> (x*y=w925:dbl)
            n365 = call "Package stage data to cluster.vi"("error in (no error)"=w927, "Increasement"=w925, "axis"=u32 4, "direction"=FALSE ("Direction")) -> ("error out"=w926:errorcluster, "Stage Ctrl"=w923:T18)  [unwired: 5 in]
          }
          frame "EPI++" {
            n366 = local read "MicroStage+"() -> (w936:dbl)
            n367 = Multiply(x=10.0, y=w936) -> (x*y=w933:dbl)
            n368 = call "Package stage data to cluster.vi"("error in (no error)"=w935, "Increasement"=w933, "axis"=u32 4, "direction"=TRUE ("Direction")) -> ("error out"=w934:errorcluster, "Stage Ctrl"=w931:T18)  [unwired: 5 in]
          }
          frame "EPI+" {
            n369 = local read "MicroStage+"() -> (w944:dbl)
            n370 = Multiply(x=1.0, y=w944) -> (x*y=w941:dbl)
            n371 = call "Package stage data to cluster.vi"("error in (no error)"=w943, "Increasement"=w941, "axis"=u32 4, "direction"=TRUE ("Direction")) -> ("error out"=w942:errorcluster, "Stage Ctrl"=w939:T18)  [unwired: 5 in]
          }
        }
        n372 = call-poly "Enqueue Message.vi"("error in (no error)"=w820, "Message Data"=w816, "Message"="StageControlChange", "Message Queue"=w815) -> ("error out"=w819:errorcluster)  [unwired: 6 in, 1 out]
      }
      frame "TIRF-LockCalbrate" {
        # "Duplicate this frame when creating new messages.  Change this comment in the duplicated frame to describe this message."
        n373 = call-poly "Enqueue Message.vi"("error in (no error)"=w947, "Message"="TIRF-LockCalbrate", "Message Queue"=w946) -> ("error out"=w950:errorcluster)  [unwired: 7 in, 1 out]
      }
      frame "TIRF-LockCalbrate Finish" {
        # "Stop - Enable/Disable buttons appropriately for an acquisition that has stopped, and update status display."
        n374 = Variant To Data(error in=w959, type=w956, Variant=w957) -> (data=w955:T2, error out=w958:errorcluster)
        n375 = Unbundle By Name(w955) -> ("Hardware Configuration.Stages Configuration.SettingValues.TirfLock.Calbrate"=w954:dbl)
        n376 = Bundle By Name(cluster=w956, "Hardware Configuration.Stages Configuration.SettingValues.TirfLock.Calbrate"=w954) -> (w953:T2)
        n377 = global write "Global.vi" "TIRF-LockIsCalbrated?"(TRUE ("TIRF-LockIsCalbrated?")) -> ()
        n378 = call "Set All Controls Status.vi"("String"="TIRF-LockCalbrated", "UI Refs"=w961, "Config"=w953) -> ()  [unwired: 9 in]
      }
      frame Default {
        # "'Default' case only runs if there is a message that isn't defined in any of the other cases.  Output a programming error."
        n379 = xnode "Error Ring"("parameter 0"=w965) -> ("error out"=w964:errorcluster)
      }
    }
    n380 = call "Error Handler - Message Handling Loop.vi"("error in (no error)"=w331, "Message Queue"=w330) -> ("dup error in"=w332:errorcluster)  [unwired: 8 in, 1 out]
  }
  n381 = Release Queue(queue=w23, error in (no error)=w48) -> (error out=w34:errorcluster)  [unwired: 1 in, 2 out]
  n382 = call "Release Data Queues.vi"("error in (no error)"=w34, "DataQueuesAndNotifier"=w21) -> ("error out"=w13:errorcluster)  [unwired: 6 in]
  n383 = Unregister For Events(event registration refnum=w44, error in=w47) -> (error out=w45:errorcluster)
  n384 = call "Release Hardware References.vi"("error in (no error)"=w13, "Config In"=w14) -> ("error out"=w12:errorcluster)  [unwired: 9 in]
  n385 = Merge Errors(w45, w12, w18, w19, w20) -> (w41:errorcluster)
  n386 = call "Destroy User Event - Stop.vi"("error in (no error)"=w41, "User Event - Stop"=w38) -> ("error out"=w40:errorcluster)  [unwired: 9 in]
  n387 = disable-structure shown="RUN_TIME_ENGINE==True" {
    disable-tunnel: w40 -> [_ _]
    frame condition #0 (active) {
    }
    frame condition #1 {
      # "Call Quit LabVIEW if running as a built application."
      n388 = Quit LabVIEW() -> ()  [unwired: 1 in]
    }
  }
  "LiveLED" <- FALSE ("Live")
  "RecordLED" <- FALSE ("Acq")
  "DeviceStatus" <- T9 {"Camera"=FALSE, "NanoStage"=FALSE, "MicroStage"=FALSE, "TIRF-Lock"=FALSE} ("DeviceStatus")
